vi "单板信息-new.vi"(8 "状态 2":string caption="系统连接状态", 11 "VIC_Receive":refnum<vi>) -> ()   [LabVIEW 2013]
panel:
  in  "偏差":dbl=10.0 format="%#.0f"
  in  "温度基准":dbl=25.0 caption="基准" format="%#.0f"
  in  "布尔 2":bool caption="判定"
  in  "偏差 2":dbl=0.05 caption="偏差" format="%.3f"
  in  "电压基准":dbl=3.7 format="%.3f"
  in  "布尔":bool caption="判定"
  out "电池充满标志位":string="是"
  out "电池运行状态":string="00"
  in  "从板板号 2":u8=1 caption="从板板号" min=1 max=30
  out "滑动杆":dbl(slide)=90.0 caption="SOC" scale=0.0..100.0 scale format="%#_6f"
  out "5":T1
  out "4":T2
  out "3":T3
  out "2":T4
  out "平均电流(A)":dbl
  out "外总压(V)":dbl
  out "总电流(A)":dbl
  out "协议是否公开":string="是"
  out "波特率":string="500Kbps"
  out "应用类型":string
  out "协议版本号":string
  out "SOH":dbl(slide)=30.0 scale=0.0..100.0 scale format="%#_6f"
  in  "刷新":bool
  in  "布尔 3":bool
  out "故障信息":string
  out "最小内阻位置":i32
  out "最大内阻位置":i32
  out "最小内阻":dbl
  out "最大内阻":dbl
  out "最低温度位置":i32
  out "最高温度位置":i32
  out "最低温度":dbl
  out "最高温度":dbl
  out "最低电压位置":i32
  out "最高电压位置":i32
  out "最低电压":dbl
  out "最高电压":dbl
  in  "主界面选项":enum32{"单选选项1", "单选选项2", "单选选项2 2"}(radio)
  in  "继电器状态 2":string[][](table)=[["RL1_ST", "", "RL5_ST"], ["RL2_ST", "", "RL6_ST"], ["RL3_ST", "", "RL7_ST"], ["RL4_ST", "", "RL8_ST"]]
  out "快换帧":T5
  out "从板参数":T6={"总电压"=0.0, "总电流"=0.0, "外总压"=0.0, "平均电流"=0.0, "SOC"=60.0, "SOH"=60.0, "最高电压"=0.0, "位置"=0.0, "最低电压"=0.0, "位置"=0.0, "压差"=0.0, "最高温度"=0.0, "位置"=0.0, "最低温度"=0.0, "位置"=0.0, "最大内阻"=0.0, "位置"=0.0, "最小内阻"=0.0, "位置"=0.0, "故障信息"="", "协议版本号"="", "应用类型"="", "波特率"="", "协议是否公开"="", "电池运行状态"="", "电池充满标志位"="", "Life:"=25.0} {"SOH" scale=0.0..100.0 scale format="%#.0f"; "SOC" scale=0.0..100.0 scale format="%#.0f"}
  out "Life:":dbl=25.0
  out "状态":bool
  out "高压板参数":T7={"总电压"=0.0, "总电流"=0.0, "外总压"=0.0, "平均电流"=0.0, "功率"=0.0, "总充电安时"=0.0, "总放电安时"=0.0, "故障信息"="", "协议版本号"="", "应用类型"="", "波特率"="", "协议是否公开"="", "电池运行状态"="", "Life:"=25.0, "正绝缘电阻"=0.0, "负绝缘电阻"=0.0} {"负绝缘电阻" format="%#.0f"; "正绝缘电阻" format="%#.0f"; "总放电安时" format="%#.0f"; "总充电安时" format="%#.0f"}
  out "继电器颜色":u32[](array[colorbox])
  out "继电器状态":string[](array[string])
  in  "选项卡控件":enum32{"从板监控", "从板信息2", "电压温度", "高压板监控"}(tab)=enum."从板信息2"
  out "从板参数":T8={"最高电压"=0.0, "位置1"=0.0, "最低电压"=0.0, "位置2"=0.0, "压差"=0.0, "最高温度"=0.0, "位置3"=0.0, "最低温度"=0.0, "位置4"=0.0, "温差"=0.0, "最高内阻"=0.0, "位置5"=0.0, "最低内阻"=0.0, "位置6"=0.0, "故障信息"="00", "最大充电总电压"=0.0, "最大充电电流"=0.0, "充电总安时"=0.0, "SOH 2"=0.0, "RL1_ST(fan)"="", "RL2_ST(heat)"="", "RL3_ST"="", "RL4_ST"="", "RL5_ST"="", "RL6_ST"="", "RL7_ST"="", "RL8_ST"=""}
  out "总电压(V)":dbl
  out "硬件故障":string[][](array[string])
  in  "欠压":u16(ring)
  in  "过压":u16(ring)
  in  "无效":u16(ring)
  in  "故障":u16(ring)
  in  "正常":u16(ring)
  out "供电电源电压(V)":string="0"
  out "内网总线负载率":string="0"
  out "供电电源状态":u16(ring)=1
  out "Flash存储器状态":u16(ring)
  out "外部EE存储器状态":u16(ring)=1
  out "内部EE存储器状态":u16(ring)=3
  out "系统时钟状态":u16(ring)
  out "内部总电压检测模块状态":u16(ring)
  out "外部总电压检测模块状态":u16(ring)
  out "绝缘检测模块状态":u16(ring)
  out "电流模块模块状态":u16(ring)=1 caption="电流检测模块状态"
  out "电池充电均衡模块状态":u16(ring)
  out "电池放电均衡模块状态":u16(ring)=1
  out "温度模块检测状态":u16(ring)=3 caption="温度检测模块状态"
  out "电压模块检测状态":u16(ring) caption="电压检测模块状态"
  out "1":T9 {"第12串" format="%#.2f"; "第11串" format="%#.2f"; "第10串" format="%#.2f"; "第9串" format="%#.2f"; "第8串" format="%#.2f"; "第7串" format="%#.2f"; "第6串" format="%#.2f"; "第5串" format="%#.2f"; "第4串" format="%#.2f"; "第3串" format="%#.2f"; "第2串" format="%#.2f"; "第1串" format="%#.2f"}
  out "1 7":T1 {"第60串" format="%.3f"; "第59串" format="%.3f"; "第58串" format="%.3f"; "第57串" format="%.3f"; "第56串" format="%.3f"; "第55串" format="%.3f"; "第54串" format="%.3f"; "第53串" format="%.3f"; "第52串" format="%.3f"; "第51串" format="%.3f"; "第50串" format="%.3f"; "第49串" format="%.3f"}
  out "1 6":T2 {"第48串" format="%.3f"; "第47串" format="%.3f"; "第46串" format="%.3f"; "第45串" format="%.3f"; "第44串" format="%.3f"; "第43串" format="%.3f"; "第42串" format="%.3f"; "第41串" format="%.3f"; "第40串" format="%.3f"; "第39串" format="%.3f"; "第38串" format="%.3f"; "第37串" format="%.3f"}
  out "1 4":T3 {"第36串" format="%.3f"; "第35串" format="%.3f"; "第34串" format="%.3f"; "第33串" format="%.3f"; "第32串" format="%.3f"; "第31串" format="%.3f"; "第30串" format="%.3f"; "第29串" format="%.3f"; "第28串" format="%.3f"; "第27串" format="%.3f"; "第26串" format="%.3f"; "第25串" format="%.3f"}
  out "1 3":T4 {"第24串" format="%.3f"; "第23串" format="%.3f"; "第22串" format="%.3f"; "第21串" format="%.3f"; "第20串" format="%.3f"; "第19串" format="%.3f"; "第18串" format="%.3f"; "第17串" format="%.3f"; "第16串" format="%.3f"; "第15串" format="%.3f"; "第14串" format="%.3f"; "第13串" format="%.3f"}
  out "1 102":T9 {"第12串" format="%.3f"; "第11串" format="%.3f"; "第10串" format="%.3f"; "第9串" format="%.3f"; "第8串" format="%.3f"; "第7串" format="%.3f"; "第6串" format="%.3f"; "第5串" format="%.3f"; "第4串" format="%.3f"; "第3串" format="%.3f"; "第2串" format="%.3f"; "第1串" format="%.3f"}
  out "高压板监控":T10={"总电压"=0.0, "总电流"=0.0, "外总压"=0.0, "平均电流"=0.0, "功率"=0.0, "总充电安时"=0.0, "总放电安时"=0.0, "正绝缘电阻"=0.0, "负绝缘电阻"=0.0, "版本协议号"="V1.2.34", "应用类型"="纯电动", "波特率"="500Kbps", "协议是否公开"="是", "故障信息"="00", "电池运行情况"="00"}
  in  "VCI_Receive":T11 {"Rsv3" max=0 format="%x"; "Rsv2" min=101 format="%x"; "Rsv1" format="%x"; "Data8" format="%x"; "Data7" format="%x"; "Data6" format="%x"; "Data5" format="%x"; "Data4" format="%x"; "Data3" format="%x"; "Data2" format="%x"; "Data1" format="%x"; "DataLen" format="%x"; "ExternFlag" format="%x"; "RemoteFlag" format="%x"; "SendType" format="%x"; "TimeFlag" format="%x"; "TimeStamp" format="%x"; "ID" format="%x"}
  in  "停止":bool
  out "单选选项2":bool
  # "Change frame"
  # "从板继电器"
  # "图例"
  # "单体电压(V)"
  # "温度(℃)"
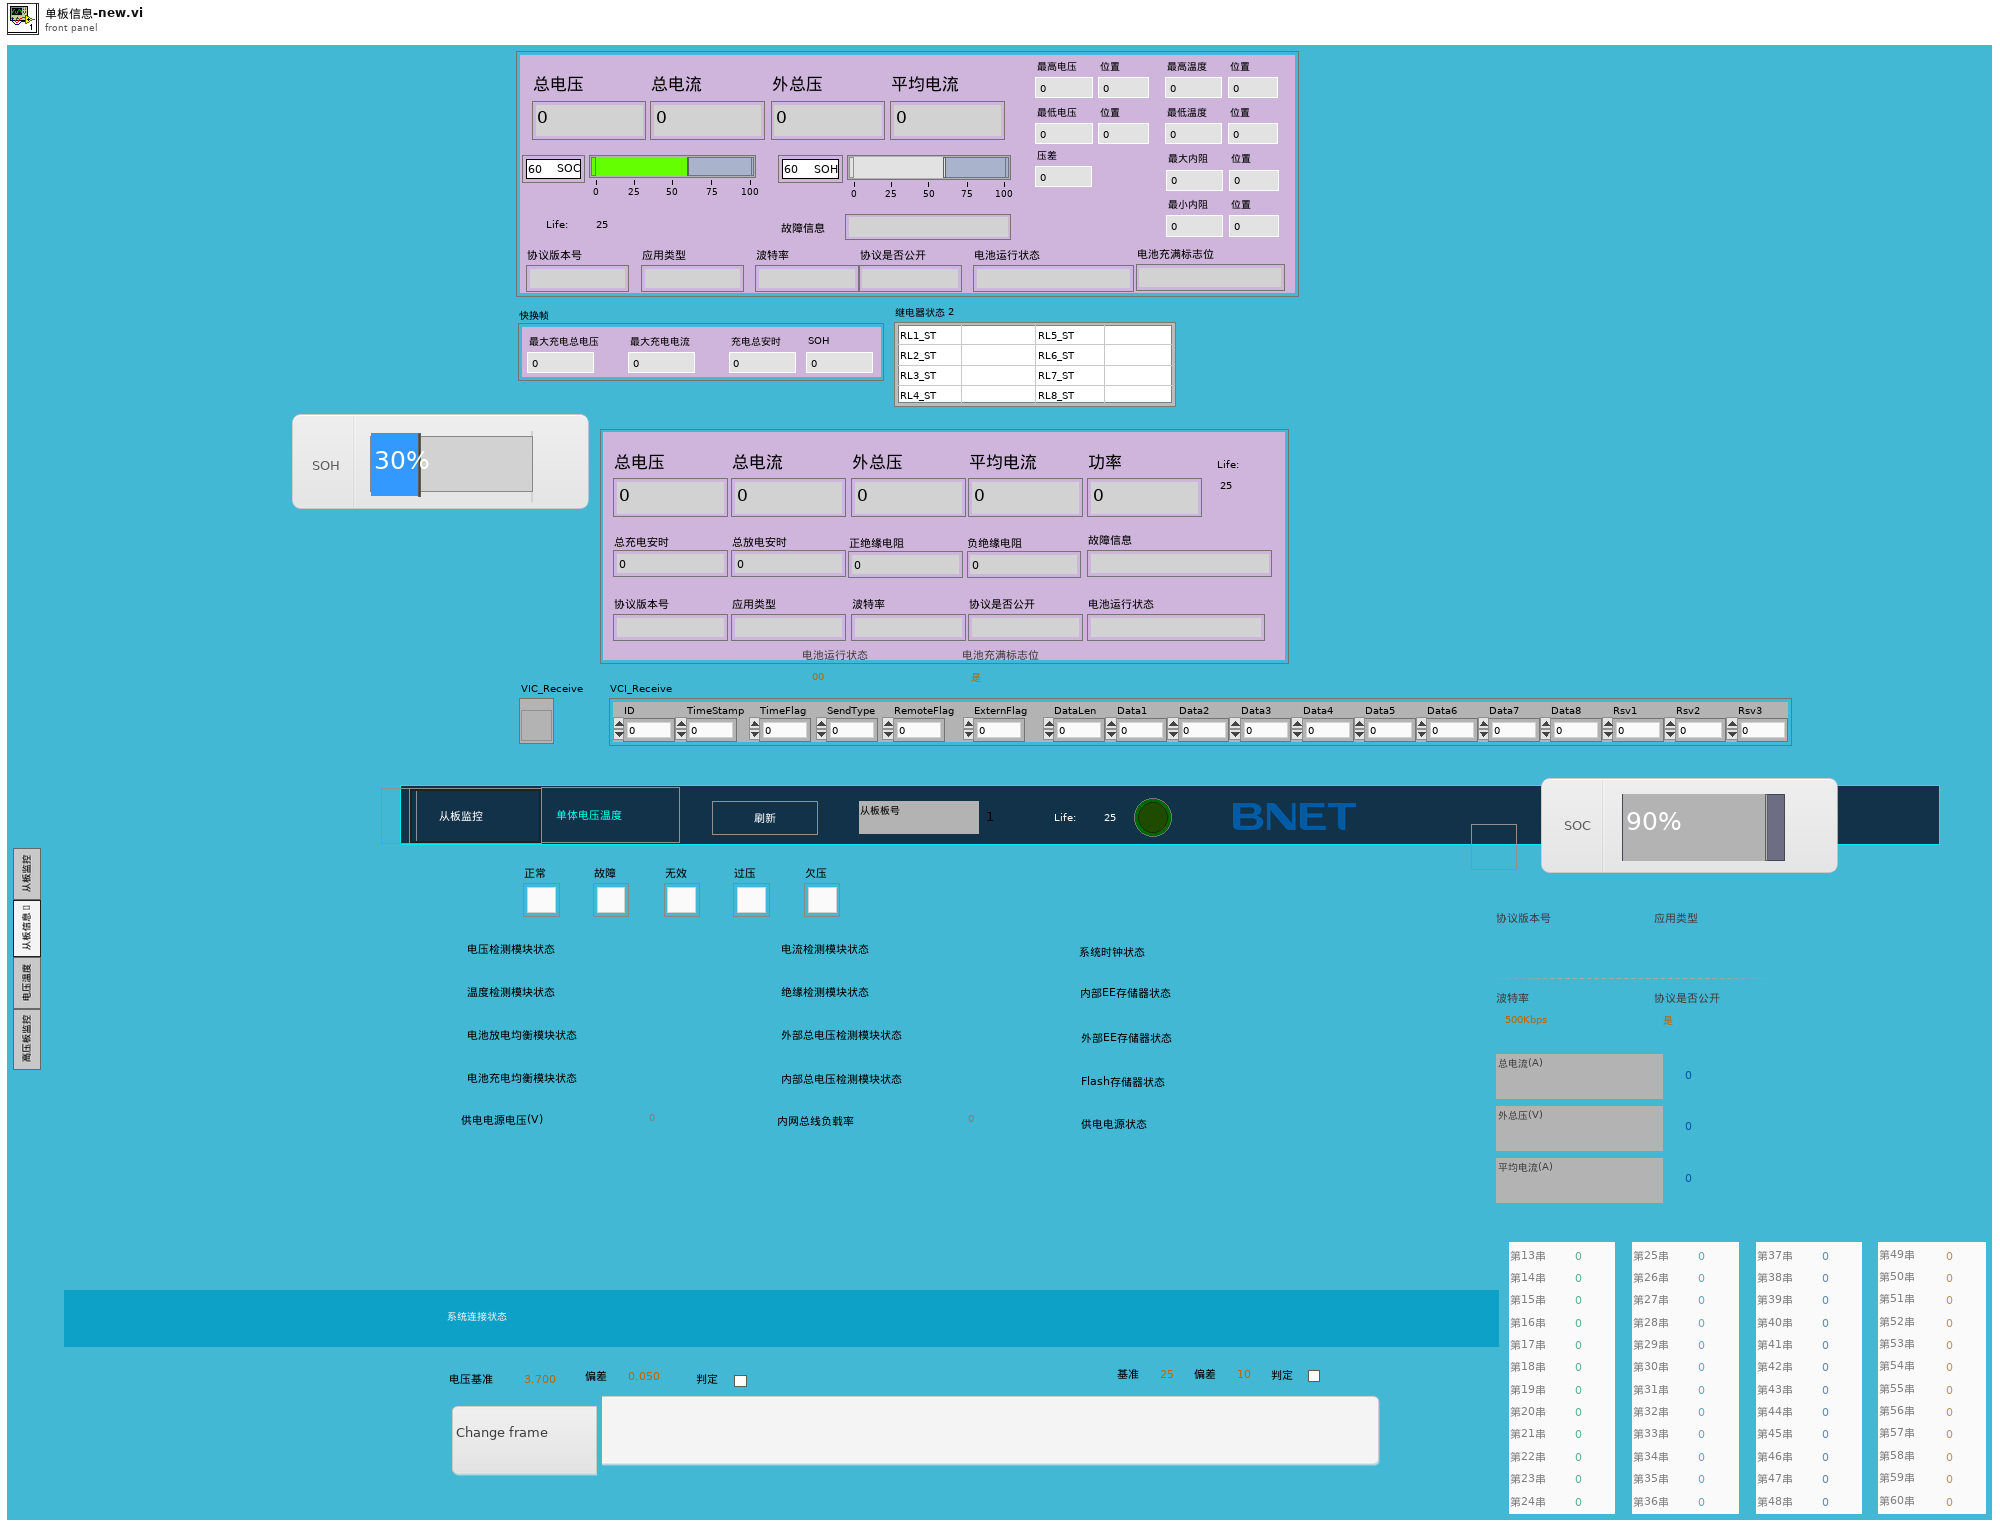
[diagram p1: front panel]
types:
  T1 = cluster{"第49串":dbl, "第50串":dbl, "第51串":dbl, "第52串":dbl, "第53串":dbl, "第54串":dbl, "第55串":dbl, "第56串":dbl, "第57串":dbl, "第58串":dbl, "第59串":dbl, "第60串":dbl}
  T2 = cluster{"第37串":dbl, "第38串":dbl, "第39串":dbl, "第40串":dbl, "第41串":dbl, "第42串":dbl, "第43串":dbl, "第44串":dbl, "第45串":dbl, "第46串":dbl, "第47串":dbl, "第48串":dbl}
  T3 = cluster{"第25串":dbl, "第26串":dbl, "第27串":dbl, "第28串":dbl, "第29串":dbl, "第30串":dbl, "第31串":dbl, "第32串":dbl, "第33串":dbl, "第34串":dbl, "第35串":dbl, "第36串":dbl}
  T4 = cluster{"第13串":dbl, "第14串":dbl, "第15串":dbl, "第16串":dbl, "第17串":dbl, "第18串":dbl, "第19串":dbl, "第20串":dbl, "第21串":dbl, "第22串":dbl, "第23串":dbl, "第24串":dbl}
  T5 = cluster{"SOH":dbl, "充电总安时":dbl, "最大充电电流":dbl, "最大充电总电压":dbl}
  T6 = cluster{"总电压":dbl, "总电流":dbl, "外总压":dbl, "平均电流":dbl, "SOC":dbl, "SOH":dbl, "最高电压":dbl, "位置":dbl, "最低电压":dbl, "位置":dbl, "压差":dbl, "最高温度":dbl, "位置":dbl, "最低温度":dbl, "位置":dbl, "最大内阻":dbl, "位置":dbl, "最小内阻":dbl, "位置":dbl, "故障信息":string, "协议版本号":string, "应用类型":string, "波特率":string, "协议是否公开":string, "电池运行状态":string, "电池充满标志位":string, "Life:":dbl}
  T7 = cluster{"总电压":dbl, "总电流":dbl, "外总压":dbl, "平均电流":dbl, "功率":dbl, "总充电安时":dbl, "总放电安时":dbl, "故障信息":string, "协议版本号":string, "应用类型":string, "波特率":string, "协议是否公开":string, "电池运行状态":string, "Life:":dbl, "正绝缘电阻":dbl, "负绝缘电阻":dbl}
  T8 = cluster{"最高电压":dbl, "位置1":dbl, "最低电压":dbl, "位置2":dbl, "压差":dbl, "最高温度":dbl, "位置3":dbl, "最低温度":dbl, "位置4":dbl, "温差":dbl, "最高内阻":dbl, "位置5":dbl, "最低内阻":dbl, "位置6":dbl, "故障信息":string, "最大充电总电压":dbl, "最大充电电流":dbl, "充电总安时":dbl, "SOH 2":dbl, "RL1_ST(fan)":string, "RL2_ST(heat)":string, "RL3_ST":string, "RL4_ST":string, "RL5_ST":string, "RL6_ST":string, "RL7_ST":string, "RL8_ST":string}
  T9 = cluster{"第1串":dbl, "第2串":dbl, "第3串":dbl, "第4串":dbl, "第5串":dbl, "第6串":dbl, "第7串":dbl, "第8串":dbl, "第9串":dbl, "第10串":dbl, "第11串":dbl, "第12串":dbl}
  T10 = cluster{"总电压":dbl, "总电流":dbl, "外总压":dbl, "平均电流":dbl, "功率":dbl, "总充电安时":dbl, "总放电安时":dbl, "正绝缘电阻":dbl, "负绝缘电阻":dbl, "版本协议号":string, "应用类型":string, "波特率":string, "协议是否公开":string, "故障信息":string, "电池运行情况":string}
  T11 = cluster{"ID":u32, "TimeStamp":u32, "TimeFlag":u8, "SendType":u8, "RemoteFlag":u8, "ExternFlag":u8, "DataLen":u8, "Data1":u8, "Data2":u8, "Data3":u8, "Data4":u8, "Data5":u8, "Data6":u8, "Data7":u8, "Data8":u8, "Rsv1":u8, "Rsv2":u8, "Rsv3":u8}
  T12 = cluster{dbl, dbl, dbl, dbl, dbl, dbl, dbl, dbl, dbl, dbl, dbl, dbl, dbl, dbl, "故障信息":string, dbl, dbl, dbl, dbl, "RL1_ST":string, "RL2_ST":string, "RL3_ST":string, "RL4_ST":string, "RL5_ST":string, "RL6_ST":string, "RL7_ST":string, "RL8_ST":string}
  T13 = enum32{"Invalid", "Standard", "Closed", "Hidden", "Minimized", "Maximized"}
  T14 = cluster{"[0]":u8, "[1]":u8, "[2]":u8, "[3]":u8, "[4]":u8, "[5]":u8, "[6]":u8, "[7]":u8, "[8]":u8, "[9]":u8, "[10]":u8, "[11]":u8}
  T15 = cluster{"[0]":dbl, "[1]":dbl, "[2]":dbl, "[3]":dbl, "[4]":dbl, "[5]":dbl, "[6]":dbl, "[7]":dbl, "[8]":dbl, "[9]":dbl, "[10]":dbl, "[11]":dbl}
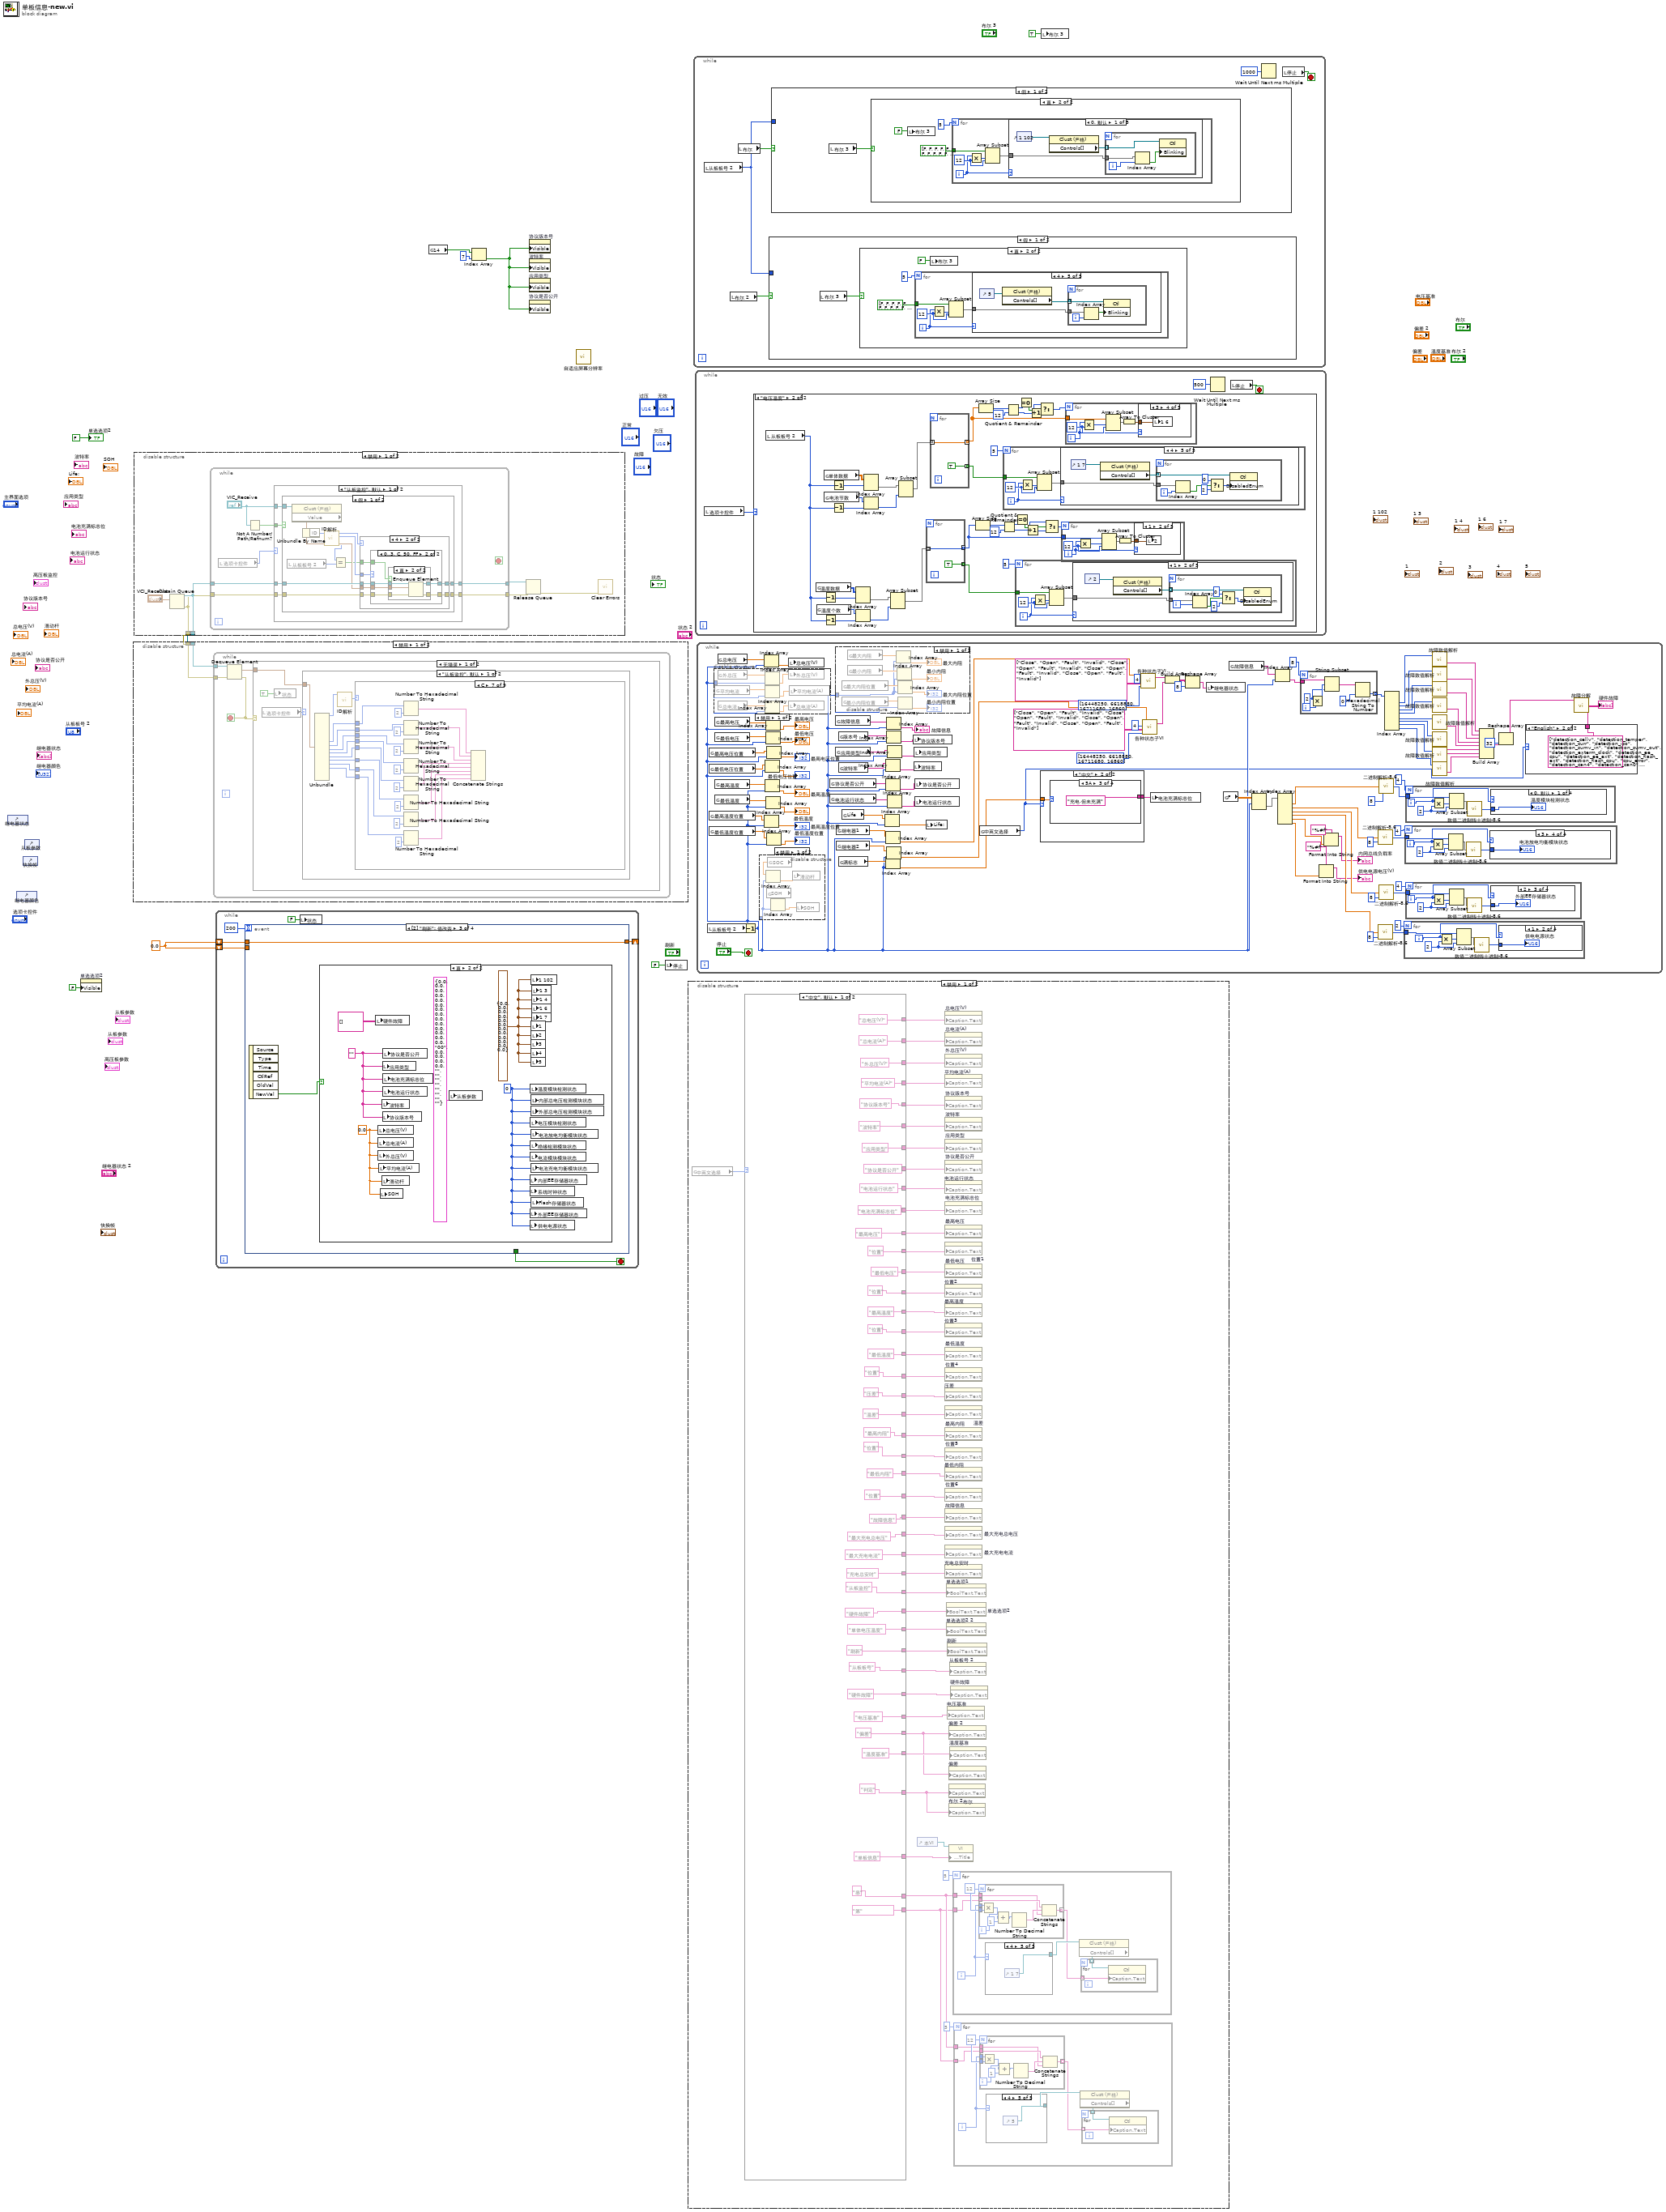
[diagram p0: block diagram]
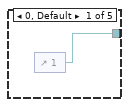
[diagram p2: hidden frame]
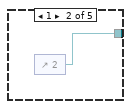
[diagram p3: hidden frame]
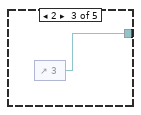
[diagram p4: hidden frame]
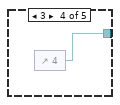
[diagram p5: hidden frame]
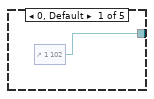
[diagram p6: hidden frame]
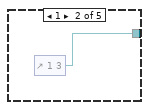
[diagram p7: hidden frame]
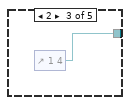
[diagram p8: hidden frame]
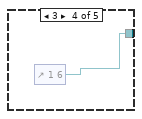
[diagram p9: hidden frame]
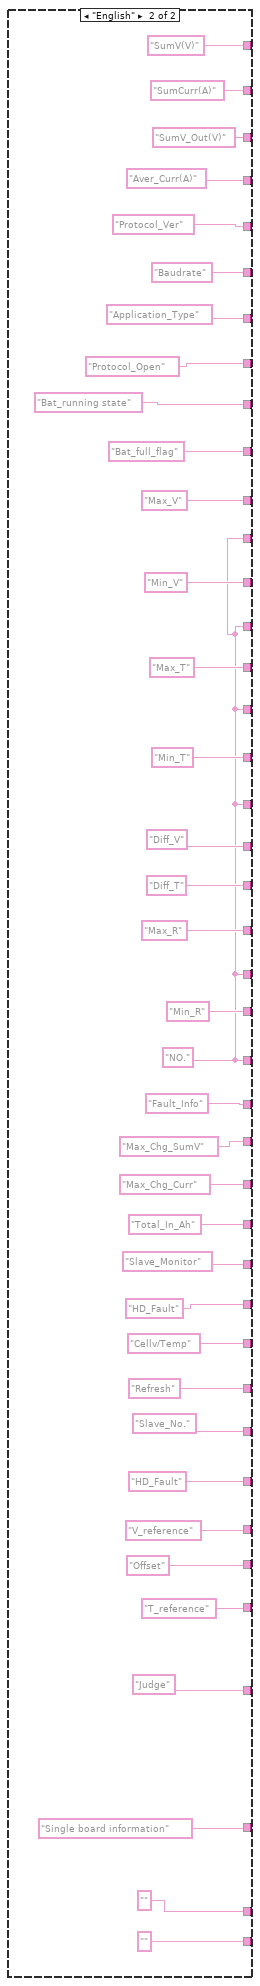
[diagram p10: hidden frame]
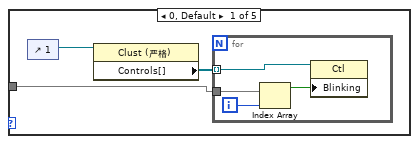
[diagram p13: hidden frame]
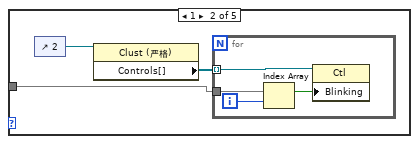
[diagram p14: hidden frame]
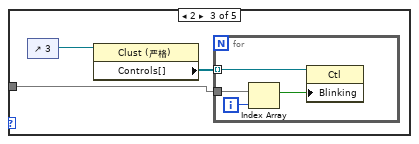
[diagram p15: hidden frame]
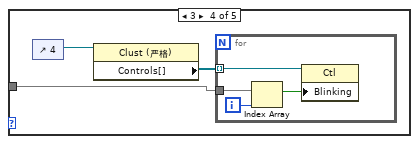
[diagram p16: hidden frame]
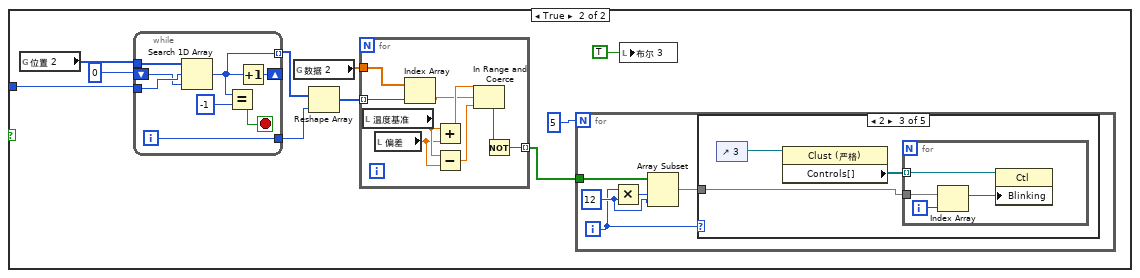
[diagram p17: hidden frame]
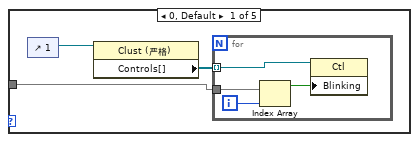
[diagram p18: hidden frame]
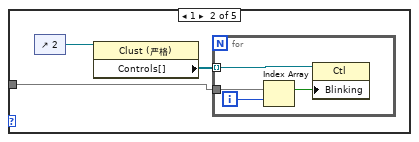
[diagram p19: hidden frame]
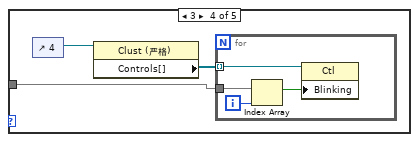
[diagram p20: hidden frame]
diagram:
  w5 = 0.0 ("Life:")
  n1 = control-ref of="继电器状态"() -> ()  [unwired: 1 out]
  n2 = control-ref of="继电器颜色"() -> ()  [unwired: 1 out]
  n3 = control-ref of="快换帧"() -> ()  [unwired: 1 out]
  n4 = control-ref of="从板参数"() -> ()  [unwired: 1 out]
  n5 = property on="单选选项2" class="Bool (严格)"("Visible"=FALSE ("可见")) -> ()  [unwired: 2 in, 2 out]
  n6 = disable-structure shown="禁用" {
    disable-tunnel: [w15 _] -> w10
    disable-tunnel: [w14 _] -> w9
    frame Disabled {
      n7 = Obtain Queue(element data type="VCI_Receive") -> (queue out=w15:refnum<queue>, error out=w14:errorcluster)  [unwired: 4 in, 1 out]
      n8 = while {
        tunnel: w15 -> [w22]
        tunnel: w14 -> [w21]
        tunnel: [w20] -> w13
        tunnel: [w19] -> w12
        stop <- w23 stop-if-true
        n9 = local read "选项卡控件"() -> (w17:enum32{"从板监控", "从板信息2", "电压温度", "高压板监控"})
        n10 = Not A Number/Path/Refnum?(number/path/refnum="VIC_Receive") -> (NaN/Path/Refnum?=w18:bool)
        n11 = case shown="\"从板监控\", 默认" w17 {
          tunnel: "VIC_Receive" -> [w30 w75]
          tunnel: w22 -> [w29 w74]
          tunnel: w21 -> [w28 w73]
          tunnel: [w27 w72] -> w20
          tunnel: [w26 w71] -> w19
          tunnel: w18 -> [w25 w70]
          frame "从板监控", Default {
            n12 = case shown="假" w25 {
              tunnel: w29 -> [w41 w69]
              tunnel: w28 -> [w40 w68]
              tunnel: [w38 w69] -> w27
              tunnel: [w37 w68] -> w26
              tunnel: w30 -> [w36 _]
              frame False {
                n13 = local read "从板板号 2"() -> (w31:u8)
                n14 = property class="Clust (严格)"(reference=w36) -> ("Value"=w39:T11)  [unwired: 1 in, 2 out]
                n15 = Unbundle By Name(w39) -> ("ID"=w42:u32)
                n16 = call "ID解析.vi"("ID"=w42) -> ("SA(4)"=w33:i32, "PF(2)"=w34:i32, "PDU(1)"=w35:i32)  [unwired: 8 out]
                n17 = Equal?(x=w33, y=w31) -> (x = y?=w32:bool)
                n18 = case shown="4" w35 {
                  tunnel: w41 -> [w44 w51]
                  tunnel: w40 -> [w43 w50]
                  tunnel: w39 -> [_ w49]
                  tunnel: [w44 w48] -> w38
                  tunnel: [w43 w47] -> w37
                  tunnel: w34 -> [_ w46]
                  tunnel: w32 -> [_ w45]
                  frame 0, Default {
                  }
                  frame 4 {
                    n19 = case shown="0..3, C, 50, FF" w46 {
                      tunnel: w51 -> [w53 w59]
                      tunnel: w50 -> [w52 w58]
                      tunnel: w49 -> [_ w57]
                      tunnel: [w53 w56] -> w48
                      tunnel: [w52 w55] -> w47
                      tunnel: w45 -> [_ w54]
                      frame 153, Default {
                      }
                      frame 0..3, 12, 80, 255 {
                        n20 = case shown="真" w54 {
                          tunnel: w59 -> [w61 w66]
                          tunnel: w58 -> [w60 w65]
                          tunnel: w57 -> [_ w64]
                          tunnel: [w61 w63] -> w56
                          tunnel: [w60 w62] -> w55
                          frame False {
                          }
                          frame True {
                            n21 = Enqueue Element(queue=w66, element=w64, error in (no error)=w65) -> (queue out=w63:refnum<queue>, error out=w62:errorcluster)  [unwired: 2 out]
                          }
                        }
                      }
                    }
                  }
                }
              }
              frame True {
                n22 = Wait Until Next ms Multiple(millisecond multiple=u32 100 ("毫秒倍数")) -> ()  [unwired: 1 out]
              }
            }
          }
          frame "高压板监控" {
            n23 = case shown="假" w70 {
              tunnel: w74 -> [w87 w115]
              tunnel: w73 -> [w86 w114]
              tunnel: [w84 w115] -> w72
              tunnel: [w83 w114] -> w71
              tunnel: w75 -> [w82 _]
              frame False {
                n24 = property class="Clust (严格)"(reference=w82) -> ("Value"=w85:T11)  [unwired: 1 in, 2 out]
                n25 = Unbundle By Name(w85) -> ("ID"=w88:u32)
                n26 = call "ID解析.vi"("ID"=w88) -> ("SA(4)"=w79:i32, "PF(2)"=w80:i32, "PDU(1)"=w81:i32)  [unwired: 8 out]
                n27 = Equal?(x=w79, y=62) -> (x = y?=w78:bool)
                n28 = case shown="4" w81 {
                  tunnel: w87 -> [w90 w97]
                  tunnel: w86 -> [w89 w96]
                  tunnel: w85 -> [_ w95]
                  tunnel: [w90 w94] -> w84
                  tunnel: [w89 w93] -> w83
                  tunnel: w80 -> [_ w92]
                  tunnel: w78 -> [_ w91]
                  frame 0, Default {
                  }
                  frame 4 {
                    n29 = case shown="0, 5, 8, C, FF" w92 {
                      tunnel: w97 -> [w99 w105]
                      tunnel: w96 -> [w98 w104]
                      tunnel: w95 -> [_ w103]
                      tunnel: [w99 w102] -> w94
                      tunnel: [w98 w101] -> w93
                      tunnel: w91 -> [_ w100]
                      frame 153, Default {
                      }
                      frame 0, 5, 8, 12, 255 {
                        n30 = case shown="真" w100 {
                          tunnel: w105 -> [w107 w112]
                          tunnel: w104 -> [w106 w111]
                          tunnel: w103 -> [_ w110]
                          tunnel: [w107 w109] -> w102
                          tunnel: [w106 w108] -> w101
                          frame False {
                          }
                          frame True {
                            n31 = Enqueue Element(queue=w112, element=w110, error in (no error)=w111) -> (queue out=w109:refnum<queue>, error out=w108:errorcluster)  [unwired: 2 out]
                          }
                        }
                      }
                    }
                  }
                }
                n32 = local write "状态"(FALSE ("接收")) -> ()
              }
              frame True {
                n33 = Wait Until Next ms Multiple(millisecond multiple=u32 100 ("毫秒倍数")) -> ()  [unwired: 1 out]
              }
            }
          }
        }
      }
      n34 = Release Queue(queue=w13, error in (no error)=w12) -> (error out=w11:errorcluster)  [unwired: 3 out]
      n35 = call <vilib>:"Clear Errors.vi"("error in (no error)"=w11) -> ()  [unwired: 7 out]
    }
    frame Enabled {
    }
  }
  n36 = disable-structure shown="禁用" {
    disable-tunnel: w10 -> [w117 _]
    disable-tunnel: w9 -> [w116 _]
    frame Disabled {
      n37 = while {
        tunnel: w117 -> [w120]
        tunnel: w116 -> [w119]
        stop <- w121 stop-if-true
        n38 = Dequeue Element(queue=w120, error in (no error)=w119) -> (element=w118:T11, error out=w121:errorcluster)  [unwired: 3 out]
        n39 = case shown="无错误" w121 {
          tunnel: w118 -> [w124 _]
          frame No Error {
            n40 = local read "选项卡控件"() -> (w123:enum32{"从板监控", "从板信息2", "电压温度", "高压板监控"})
            n41 = local write "状态"(TRUE ("接收")) -> ()
            n42 = case shown="\"从板监控\", 默认" w123 {
              tunnel: w124 -> [w135 w321]
              frame "从板监控", Default {
                n43 = Unbundle(w135) -> ("ID"=w134:u32, "Data1"=w132:u8, "Data2"=w131:u8, "Data3"=w130:u8, "Data4"=w129:u8, "Data5"=w128:u8, "Data6"=w127:u8, "Data7"=w126:u8, "Data8"=w125:u8)  [unwired: 9 out]
                n44 = call "ID解析.vi"("ID"=w134) -> ("PF(2)"=w133:i32)  [unwired: 10 out]
                n45 = case shown="C" w133 {
                  tunnel: w132 -> [_ w145 w174 w188 w210 w242 w262 w280 w285]
                  tunnel: w131 -> [_ w144 w173 w187 w209 w241 w261 _ w284]
                  tunnel: w130 -> [_ w143 w172 w186 w208 w240 w260 _ w283]
                  tunnel: w129 -> [_ w142 w171 w185 w207 w239 w259 _ _]
                  tunnel: w128 -> [_ w141 w170 w184 w206 w238 w258 _ w282]
                  tunnel: w127 -> [_ w140 w169 w183 w205 w237 w257 w279 _]
                  tunnel: w126 -> [_ w139 w156 w182 w204 w236 w256 _ _]
                  tunnel: w125 -> [_ w138 w155 _ w203 _ w255 _ w281]
                  frame 153, Default {
                    n46 = Wait Until Next ms Multiple(millisecond multiple=u32 2 ("毫秒倍数")) -> ()  [unwired: 1 out]
                  }
                  frame 0 {
                    n47 = Join Numbers(hi=w143, lo=w142) -> ((hi.lo)=w150:u16)
                    n48 = Join Numbers(hi=w141, lo=w140) -> ((hi.lo)=w152:u16)
                    n49 = Join Numbers(hi=w145, lo=w144) -> ((hi.lo)=w151:u16)
                    n50 = Join Numbers(hi=w139, lo=w138) -> ((hi.lo)=w146:u16)
                    n51 = call "输出分辨率计算.vi"("偏移量"=sgl -3000.0, "分辨率"=0.1, "数值 3"=w150, "数值 2"=w146) -> ()  [unwired: 2 in, 6 out]
                    n52 = call "输出分辨率计算.vi"("分辨率"=0.1, "数值 3"=w152, "数值 2"=w151) -> ("输出2"=w137:dbl)  [unwired: 3 in, 5 out]
                  }
                  frame 144 {
                    n53 = Join Numbers(hi=w172, lo=w171) -> ((hi.lo)=w178:u16)
                    n54 = Join Numbers(hi=w170, lo=w169) -> ((hi.lo)=w168:u16)
                    n55 = Join Numbers(hi=w174, lo=w173) -> ((hi.lo)=w179:u16)
                    n56 = call "二进制解析-8.6.vi"("索引"=8, "数值"=w156) -> ("低位子数组"=w159:i32[])  [unwired: 3 out]
                    n57 = call "二进制解析-8.6.vi"("索引"=4, "数值"=w155) -> ("高位子数组"=w158:i32[])  [unwired: 3 out]
                    n58 = Insert Into Array(array=w159, new element=w158) -> (w157:i32[])  [unwired: 1 in]
                    n59 = call "输出分辨率计算.vi"("分辨率"=0.001, "数值 2"=w168) -> ("输出2"=w162:dbl)  [unwired: 4 in, 5 out]
                    n60 = local read "快换帧"() -> (w166:T5)
                    n61 = call "数值二进制转十进制-8.6.vi"("子数组"=w157) -> ("十进制数值"=w154:i32)  [unwired: 4 out]
                    n62 = call "输出分辨率计算.vi"("分辨率"=0.1, "数值 3"=w154, "数值 2"=w179) -> ("输出3"=w153:dbl, "输出2"=w163:dbl)  [unwired: 3 in, 4 out]
                    n63 = call "输出分辨率计算.vi"("偏移量"=sgl -3000.0, "分辨率"=0.1, "数值 3"=w178) -> ("输出3"=w164:dbl)  [unwired: 3 in, 5 out]
                    n64 = Bundle(cluster=w166, "SOH"=w153, "充电总安时"=w162, "最大充电电流"=w164, "最大充电总电压"=w163) -> (w165:T5)
                    n65 = local write "快换帧"(w165) -> ()
                  }
                  frame 1 {
                    n66 = Join Numbers(hi=w188, lo=w187) -> ((hi.lo)=w189:u16)
                    n67 = Join Numbers(hi=w186, lo=w185) -> ((hi.lo)=w190:u16)
                    n68 = call "二进制解析-8.6.vi"("索引"=8, "数值"=w182) -> ("低位子数组"=w198:i32[])  [unwired: 3 out]
                    n69 = call "二进制解析-8.6.vi"("索引"=8, "数值"=w184) -> ("低位子数组"=w195:i32[])  [unwired: 3 out]
                    n70 = call "二进制解析-8.6.vi"("索引"=4, "数值"=w183) -> ("低位子数组"=w197:i32[], "高位子数组"=w196:i32[])  [unwired: 2 out]
                    n71 = Insert Into Array(array=w195, new element=w196) -> (w200:i32[])  [unwired: 1 in]
                    n72 = Insert Into Array(array=w197, new element=w198) -> (w199:i32[])  [unwired: 1 in]
                    n73 = call "输出分辨率计算.vi"("分辨率"=0.001, "数值 3"=w190, "数值 2"=w189) -> ("输出3"=w181:dbl, "输出2"=w180:dbl)  [unwired: 3 in, 4 out]
                    n74 = call "数值二进制转十进制-8.6.vi"("子数组"=w200) -> ()  [unwired: 5 out]
                    n75 = call "数值二进制转十进制-8.6.vi"("子数组"=w199) -> ()  [unwired: 5 out]
                  }
                  frame 2 {
                    n76 = call "二进制解析-8.6.vi"("索引"=8, "数值"=w203) -> ("低位子数组"=w224:i32[])  [unwired: 3 out]
                    n77 = call "二进制解析-8.6.vi"("索引"=8, "数值"=w205) -> ("低位子数组"=w227:i32[])  [unwired: 3 out]
                    n78 = call "二进制解析-8.6.vi"("索引"=4, "数值"=w204) -> ("低位子数组"=w225:i32[], "高位子数组"=w226:i32[])  [unwired: 2 out]
                    n79 = call "二进制解析-8.6.vi"("索引"=8, "数值"=w206) -> ("低位子数组"=w218:i32[])  [unwired: 3 out]
                    n80 = call "二进制解析-8.6.vi"("索引"=8, "数值"=w208) -> ("低位子数组"=w215:i32[])  [unwired: 3 out]
                    n81 = call "二进制解析-8.6.vi"("索引"=4, "数值"=w207) -> ("低位子数组"=w217:i32[], "高位子数组"=w216:i32[])  [unwired: 2 out]
                    n82 = call "输出分辨率计算.vi"("偏移量"=sgl -40.0, "分辨率"=1.0, "数值 3"=w209, "数值 2"=w210) -> ()  [unwired: 2 in, 6 out]
                    n83 = Insert Into Array(array=w227, new element=w226) -> (w222:i32[])  [unwired: 1 in]
                    n84 = Insert Into Array(array=w225, new element=w224) -> (w223:i32[])  [unwired: 1 in]
                    n85 = Insert Into Array(array=w215, new element=w216) -> (w220:i32[])  [unwired: 1 in]
                    n86 = Insert Into Array(array=w217, new element=w218) -> (w219:i32[])  [unwired: 1 in]
                    n87 = call "数值二进制转十进制-8.6.vi"("子数组"=w222) -> ("十进制数值"=w231:i32)  [unwired: 4 out]
                    n88 = call "数值二进制转十进制-8.6.vi"("子数组"=w220) -> ()  [unwired: 5 out]
                    n89 = call "数值二进制转十进制-8.6.vi"("子数组"=w223) -> ("十进制数值"=w232:i32)  [unwired: 4 out]
                    n90 = call "数值二进制转十进制-8.6.vi"("子数组"=w219) -> ()  [unwired: 5 out]
                    n91 = call "输出分辨率计算.vi"("分辨率"=0.1, "数值 3"=w232, "数值 2"=w231) -> ("输出3"=w201:dbl, "输出2"=w202:dbl)  [unwired: 3 in, 4 out]
                  }
                  frame 3 {
                    n92 = Join Numbers(hi=w242, lo=w241) -> ((hi.lo)=w243:u16)
                    n93 = Join Numbers(hi=w240, lo=w239) -> ((hi.lo)=w244:u16)
                    n94 = call "二进制解析-8.6.vi"("索引"=8, "数值"=w236) -> ("低位子数组"=w252:i32[])  [unwired: 3 out]
                    n95 = call "二进制解析-8.6.vi"("索引"=8, "数值"=w238) -> ("低位子数组"=w249:i32[])  [unwired: 3 out]
                    n96 = call "二进制解析-8.6.vi"("索引"=4, "数值"=w237) -> ("低位子数组"=w251:i32[], "高位子数组"=w250:i32[])  [unwired: 2 out]
                    n97 = Insert Into Array(array=w249, new element=w250) -> (w254:i32[])  [unwired: 1 in]
                    n98 = Insert Into Array(array=w251, new element=w252) -> (w253:i32[])  [unwired: 1 in]
                    n99 = call "输出分辨率计算.vi"("分辨率"=0.001, "数值 3"=w244, "数值 2"=w243) -> ("输出3"=w234:dbl, "输出2"=w235:dbl)  [unwired: 3 in, 4 out]
                    n100 = call "数值二进制转十进制-8.6.vi"("子数组"=w254) -> ()  [unwired: 5 out]
                    n101 = call "数值二进制转十进制-8.6.vi"("子数组"=w253) -> ()  [unwired: 5 out]
                  }
                  frame 12 {
                    n102 = Number To Hexadecimal String(1:i16 2 ("宽度(-)"), 2:w262) -> (0:w271:string)
                    n103 = Number To Hexadecimal String(1:i16 2 ("宽度(-)"), 2:w261) -> (0:w272:string)
                    n104 = Number To Hexadecimal String(1:i16 2 ("宽度(-)"), 2:w260) -> (0:w273:string)
                    n105 = Number To Hexadecimal String(1:i16 2 ("宽度(-)"), 2:w259) -> (0:w274:string)
                    n106 = Number To Hexadecimal String(1:i16 2 ("宽度(-)"), 2:w258) -> (0:w275:string)
                    n107 = Number To Hexadecimal String(1:i16 2 ("宽度(-)"), 2:w257) -> (0:w276:string)
                    n108 = Number To Hexadecimal String(1:i16 2 ("宽度(-)"), 2:w256) -> (0:w277:string)
                    n109 = Number To Hexadecimal String(1:i16 2 ("宽度(-)"), 2:w255) -> (0:w278:string)
                    n110 = Concatenate Strings(w271, w272, w273, w274, w275, w276, w277, w278) -> ()  [unwired: 1 out]
                  }
                  frame 80 {
                  }
                  frame 255 {
                    n111 = call "二进制解析-8.6.vi"("索引"=4, "数值"=w285) -> ("低位子数组"=w286:i32[], "高位子数组"=w287:i32[])  [unwired: 2 out]
                    n112 = call "二进制解析-8.6.vi"("索引"=6, "数值"=w284) -> ("低位子数组"=w297:i32[], "高位子数组"=w296:i32[])  [unwired: 2 out]
                    n113 = call "二进制解析-8.6.vi"("索引"=7, "数值"=w283) -> ("高位子数组"=w301:i32[])  [unwired: 3 out]
                    n114 = call "数值二进制转十进制-8.6.vi"("子数组"=w297) -> ("十进制数值"=w298:i32)  [unwired: 4 out]
                    n115 = call "数值二进制转十进制-8.6.vi"("子数组"=w286) -> ("十进制数值"=w289:i32)  [unwired: 4 out]
                    n116 = call "数值二进制转十进制-8.6.vi"("子数组"=w296) -> ("十进制数值"=w299:i32)  [unwired: 4 out]
                    n117 = call "数值二进制转十进制-8.6.vi"("子数组"=w301) -> ("十进制数值"=w302:i32)  [unwired: 4 out]
                    n118 = call "数值二进制转十进制-8.6.vi"("子数组"=w287) -> ("十进制数值"=w288:i32)  [unwired: 4 out]
                    n119 = case shown="1" w302 {
                      tunnel: ["不公开" "公开"] -> _
                      frame 0, Default {
                      }
                      frame 1 {
                      }
                    }
                    n120 = case shown="0, 默认" w298 {
                      tunnel: ["500Kps" "250Kps"] -> _
                      frame 0, Default {
                      }
                      frame 1 {
                      }
                    }
                    n121 = Number To Decimal String(number=w288) -> (decimal integer string=w290:string)  [unwired: 1 out]
                    n122 = case shown="4" w299 {
                      tunnel: [_ "纯电动BMS" "混合动力BMS" "储能" "快换"] -> _
                      frame 0, Default {
                      }
                      frame 1 {
                      }
                      frame 2 {
                      }
                      frame 3 {
                      }
                      frame 4 {
                      }
                    }
                    n123 = Number To Decimal String(number=w289) -> (decimal integer string=w292:string)  [unwired: 1 out]
                    n124 = call "运行模式解析.vi"("输入值"=w282) -> ()  [unwired: 1 in, 1 out]
                    n125 = Concatenate Strings("V" ("字符串"), w290, "." ("字符串"), w292) -> ()  [unwired: 1 out]
                  }
                }
              }
              frame "高压板监控" {
                n126 = Unbundle(w321) -> ("ID"=w320:u32, "Data1"=w318:u8, "Data2"=w317:u8, "Data3"=w316:u8, "Data4"=w315:u8, "Data5"=w314:u8, "Data6"=w313:u8, "Data7"=w312:u8, "Data8"=w311:u8)  [unwired: 9 out]
                n127 = call "ID解析.vi"("ID"=w320) -> ("PF(2)"=w319:i32)  [unwired: 10 out]
                n128 = case shown="99, 默认" w319 {
                  tunnel: w318 -> [_ w336 w355 w373 w401]
                  tunnel: w317 -> [_ w335 w354 w372 w400]
                  tunnel: w316 -> [_ w334 w353 w371 w399]
                  tunnel: w315 -> [_ w333 w352 w370 _]
                  tunnel: w314 -> [_ w332 w351 w369 w398]
                  tunnel: w313 -> [_ w331 w350 w368 _]
                  tunnel: w312 -> [_ w330 w349 w367 _]
                  tunnel: w311 -> [_ w329 w348 w366 w397]
                  frame 153, Default {
                    n129 = Wait Until Next ms Multiple(millisecond multiple=u32 2 ("毫秒倍数")) -> ()  [unwired: 1 out]
                  }
                  frame 0 {
                    n130 = Join Numbers(hi=w334, lo=w333) -> ((hi.lo)=w341:u16)
                    n131 = Join Numbers(hi=w332, lo=w331) -> ((hi.lo)=w343:u16)
                    n132 = Join Numbers(hi=w336, lo=w335) -> ((hi.lo)=w342:u16)
                    n133 = Join Numbers(hi=w330, lo=w329) -> ((hi.lo)=w337:u16)
                    n134 = call "输出分辨率计算.vi"("偏移量"=sgl -3000.0, "分辨率"=0.1, "数值 3"=w341, "数值 2"=w337) -> ("输出3"=w323:dbl, "输出2"=w324:dbl)  [unwired: 2 in, 4 out]
                    n135 = call "输出分辨率计算.vi"("分辨率"=0.1, "数值 3"=w343, "数值 2"=w342) -> ("输出3"=w325:dbl, "输出2"=w326:dbl)  [unwired: 3 in, 4 out]
                    n136 = local read "高压板监控"() -> (w328:T10)
                    n137 = Bundle By Name(cluster=w328, "总电压"=w326, "外总压"=w325, "平均电流"=w324, "总电流"=w323) -> (w327:T10)
                    n138 = local write "高压板监控"(w327) -> ()
                  }
                  frame 5 {
                    n139 = Join Numbers(hi=w355, lo=w354) -> ((hi.lo)=w358:u16)
                    n140 = Join Numbers(hi=w353, lo=w352) -> ((hi.lo)=w357:u16)
                    n141 = Join Numbers(hi=w351, lo=w350) -> ((hi.lo)=w359:u16)
                    n142 = Join Numbers(hi=w349, lo=w348) -> ((hi.lo)=w360:u16)
                    n143 = Join Numbers(hi=w358, lo=w357) -> ((hi.lo)=w362:u32)
                    n144 = Join Numbers(hi=w359, lo=w360) -> ((hi.lo)=w361:u32)
                    n145 = call "输出分辨率计算.vi"("分辨率"=0.001, "数值 3"=w361, "数值 2"=w362) -> ("输出3"=w345:dbl, "输出2"=w346:dbl)  [unwired: 3 in, 4 out]
                    n146 = local read "高压板监控"() -> (w347:T10)
                    n147 = Bundle By Name(cluster=w347, "总充电安时"=w346, "总放电安时"=w345) -> (w344:T10)
                    n148 = local write "高压板监控"(w344) -> ()
                  }
                  frame 12 {
                    n149 = Number To Hexadecimal String(1:i16 2 ("宽度(-)"), 2:w373) -> (0:w382:string)
                    n150 = Number To Hexadecimal String(1:i16 2 ("宽度(-)"), 2:w372) -> (0:w383:string)
                    n151 = Number To Hexadecimal String(1:i16 2 ("宽度(-)"), 2:w371) -> (0:w384:string)
                    n152 = Number To Hexadecimal String(1:i16 2 ("宽度(-)"), 2:w370) -> (0:w385:string)
                    n153 = Number To Hexadecimal String(1:i16 2 ("宽度(-)"), 2:w369) -> (0:w386:string)
                    n154 = Number To Hexadecimal String(1:i16 2 ("宽度(-)"), 2:w368) -> (0:w387:string)
                    n155 = Number To Hexadecimal String(1:i16 2 ("宽度(-)"), 2:w367) -> (0:w388:string)
                    n156 = Number To Hexadecimal String(1:i16 2 ("宽度(-)"), 2:w366) -> (0:w389:string)
                    n157 = Concatenate Strings(w382, w383, w384, w385, w386, w387, w388, w389) -> (w364:string)
                    n158 = local read "高压板监控"() -> (w365:T10)
                    n159 = Bundle By Name(cluster=w365, "故障信息"=w364) -> (w363:T10)
                    n160 = local write "高压板监控"(w363) -> ()
                  }
                  frame 255 {
                    n161 = local write "Life:"(w397) -> ()
                    n162 = call "二进制解析-8.6.vi"("索引"=4, "数值"=w401) -> ("低位子数组"=w402:i32[], "高位子数组"=w403:i32[])  [unwired: 2 out]
                    n163 = call "二进制解析-8.6.vi"("索引"=6, "数值"=w400) -> ("低位子数组"=w413:i32[], "高位子数组"=w412:i32[])  [unwired: 2 out]
                    n164 = call "二进制解析-8.6.vi"("索引"=7, "数值"=w399) -> ("高位子数组"=w417:i32[])  [unwired: 3 out]
                    n165 = call "数值二进制转十进制-8.6.vi"("子数组"=w413) -> ("十进制数值"=w414:i32)  [unwired: 4 out]
                    n166 = call "数值二进制转十进制-8.6.vi"("子数组"=w402) -> ("十进制数值"=w405:i32)  [unwired: 4 out]
                    n167 = call "数值二进制转十进制-8.6.vi"("子数组"=w412) -> ("十进制数值"=w415:i32)  [unwired: 4 out]
                    n168 = call "数值二进制转十进制-8.6.vi"("子数组"=w417) -> ("十进制数值"=w418:i32)  [unwired: 4 out]
                    n169 = call "数值二进制转十进制-8.6.vi"("子数组"=w403) -> ("十进制数值"=w404:i32)  [unwired: 4 out]
                    n170 = case shown="1" w418 {
                      tunnel: ["不公开" "公开"] -> w392
                      frame 0, Default {
                      }
                      frame 1 {
                      }
                    }
                    n171 = case shown="0, 默认" w414 {
                      tunnel: ["500Kps" "250Kps"] -> w393
                      frame 0, Default {
                      }
                      frame 1 {
                      }
                    }
                    n172 = Number To Decimal String(number=w404) -> (decimal integer string=w406:string)  [unwired: 1 out]
                    n173 = case shown="4" w415 {
                      tunnel: [_ "纯电动BMS" "混合动力BMS" "储能" "快换"] -> w394
                      frame 0, Default {
                      }
                      frame 1 {
                      }
                      frame 2 {
                      }
                      frame 3 {
                      }
                      frame 4 {
                      }
                    }
                    n174 = Number To Decimal String(number=w405) -> (decimal integer string=w408:string)  [unwired: 1 out]
                    n175 = call "运行模式解析.vi"("输入值"=w398) -> ("输出值"=w391:string)  [unwired: 1 in]
                    n176 = Concatenate Strings("V" ("字符串"), w406, "." ("字符串"), w408) -> (w395:string)
                    n177 = local read "高压板监控"() -> (w396:T10)
                    n178 = Bundle By Name(cluster=w396, "版本协议号"=w395, "应用类型"=w394, "波特率"=w393, "协议是否公开"=w392, "电池运行情况"=w391) -> (w390:T10)
                    n179 = local write "高压板监控"(w390) -> ()
                  }
                }
              }
            }
          }
          frame Error {
            n180 = Wait Until Next ms Multiple(millisecond multiple=u32 100 ("毫秒倍数")) -> ()  [unwired: 1 out]
          }
        }
      }
    }
    frame Enabled {
    }
  }
  n181 = while {
    shift-right: [w431] -> _
    shift-left: w5 -> [w430]
    shift-left: w5 -> [w429]
    stop <- w432 stop-if-true
    n182 = event shown="[2] \"刷新\": 值改变" {
      selector: _ -> [_ _ _ _]
      dyn-events: _ -> [_ _ _ _]
      timeout: 200 -> [_ _ _ _]
      tunnel: [_ _ _ w519] -> w432
      tunnel: [w437 w500 w511 w518] -> w431
      tunnel: w430 -> [w436 w500 w511 w518]
      tunnel: w429 -> [w435 _ _ _]
      event Timeout {
        n183 = event-data() -> ()  [unwired: 3 out]
        n184 = control-ref of="单选选项2 2"() -> (w439:refnum<vi>)
        n185 = control-ref of="单选选项2"() -> (w446:refnum<vi>)
        n186 = control-ref of="单选选项1"() -> (w447:refnum<vi>)
        n187 = local read "主界面选项"() -> (w448:enum32{"单选选项1", "单选选项2", "单选选项2 2"})
        n188 = Not Equal?(x=w436, y=w435) -> (x != y?=w434:bool)
        n189 = Build Array(w447, w446, w439) -> (w445:refnum<vi>[])
        n190 = local write "状态"(w434) -> ()
        n191 = case shown="\"单选选项2\"" w448 {
          selector: w448 -> [w483 w490 w496]
          tunnel: w445 -> [w484 w493 w499]
          tunnel: [w482 w492 w498] -> w442
          tunnel: [w481 w491 w497] -> w441
          tunnel: [TRUE TRUE TRUE] -> w440
          tunnel: [enum32{"从板监控", "从板信息2", "电压温度", "高压板监控"}."从板监控" ("选项卡控件") enum32{"从板监控", "从板信息2", "电压温度", "高压板监控"}."从板信息2" ("选项卡控件") enum32{"从板监控", "从板信息2", "电压温度", "高压板监控"}."电压温度" ("选项卡控件")] -> w438
          frame "单选选项1", Default {
            n192 = local read "继电器状态"() -> (w487:string[])
            n193 = local read "快换帧"() -> (w486:T5)
            n194 = local read "最高电压位置"() -> (w462:i32)
            n195 = local read "最低电压位置"() -> (w461:i32)
            n196 = local read "最高温度位置"() -> (w458:i32)
            n197 = local read "最低温度位置"() -> (w457:i32)
            n198 = local read "最大内阻位置"() -> (w455:i32)
            n199 = local read "最小内阻位置"() -> (w453:i32)
            n200 = local read "最高电压"() -> (w464:dbl)
            n201 = local read "最低电压"() -> (w463:dbl)
            n202 = local read "最高温度"() -> (w460:dbl)
            n203 = local read "最低温度"() -> (w459:dbl)
            n204 = local read "最大内阻"() -> (w456:dbl)
            n205 = local read "最小内阻"() -> (w454:dbl)
            n206 = local read "故障信息"() -> (w466:string)
            n207 = Index Array(array=w487) -> (element #1=w475:string, element #2=w474:string, element #3=w473:string, element #4=w472:string, element #5=w471:string, element #6=w470:string, element #7=w469:string, element #8=w468:string)  [unwired: 8 in]
            n208 = Unbundle(w486) -> ("SOH"=w451:dbl, "充电总安时"=w479:dbl, "最大充电电流"=w478:dbl, "最大充电总电压"=w477:dbl)
            n209 = Delete From Array(array=w484, index=w483) -> (deleted portion=w481:refnum<vi>, array with subset deleted=w482:refnum<vi>[])  [unwired: 1 in]
            n210 = local read "从板参数"() -> (w476:T8)
            n211 = Subtract(x=w464, y=w463) -> (x-y=w465:dbl)
            n212 = Subtract(x=w460, y=w459) -> (x-y=w480:dbl)
            n213 = Bundle(cluster=w476, "最高电压"=w464, "位置1"=w462, "最低电压"=w463, "位置2"=w461, "压差"=w465, "最高温度"=w460, "位置3"=w458, "最低温度"=w459, "位置4"=w457, "温差"=w480, "最高内阻"=w456, "位置5"=w455, "最低内阻"=w454, "位置6"=w453, "故障信息"=w466, "最大充电总电压"=w477, "最大充电电流"=w478, "充电总安时"=w479, "SOH 2"=w451, "RL1_ST(fan)"=w475, "RL2_ST(heat)"=w474, "RL3_ST"=w473, "RL4_ST"=w472, "RL5_ST"=w471, "RL6_ST"=w470, "RL7_ST"=w469, "RL8_ST"=w468) -> (w485:T8)
            n214 = local write "从板参数"(w485) -> ()
          }
          frame "单选选项2" {
            n215 = Delete From Array(array=w493, index=w490) -> (deleted portion=w491:refnum<vi>, array with subset deleted=w492:refnum<vi>[])  [unwired: 1 in]
          }
          frame "单选选项2 2" {
            n216 = Delete From Array(array=w499, index=w496) -> (deleted portion=w497:refnum<vi>, array with subset deleted=w498:refnum<vi>[])  [unwired: 1 in]
          }
        }
        n217 = for {
          tunnel: w442 -> [w450] mode=indexing
          tunnel: u32 16777215 -> [w449]
          n218 = property class="Bool (严格)"(reference=w450, "BoolText.TextColor"=w449) -> ()  [unwired: 1 in, 2 out]
        }
        n219 = property class="Bool (严格)"(reference=w441, "BoolText.TextColor"=u32 65511) -> ()  [unwired: 1 in, 2 out]
        n220 = local write "选项卡控件"(w438) -> ()
        n221 = property on="从板板号 2" class="DigNum (严格)"("Visible"=w440) -> ()  [unwired: 2 in, 2 out]
        n222 = local read "Life:"() -> (w437:dbl)
      }
      event "从板板号 2": Value Change {
        n223 = event-data() -> ("OldVal"=w503:u8, "NewVal"=w502:u8)  [unwired: 5 out]
        n224 = Not Equal?(x=w503, y=w502) -> (x != y?=w501:bool)
        n225 = case shown="真" w501 {
          frame False {
          }
          frame True {
            w504 = 0
            w506 = T9 {"第1串"=0.0, "第2串"=0.0, "第3串"=0.0, "第4串"=0.0, "第5串"=0.0, "第6串"=0.0, "第7串"=0.0, "第8串"=0.0, "第9串"=0.0, "第10串"=0.0, "第11串"=0.0, "第12串"=0.0} ("1 102")
            w508 = 0.0 ("总电压")
            w509 = "" ("协议是否公开")
            n226 = local write "硬件故障"(string[][] [] ("电池故障 2")) -> ()
            n227 = local write "总电压(V)"(w508) -> ()
            n228 = local write "总电流(A)"(w508) -> ()
            n229 = local write "外总压(V)"(w508) -> ()
            n230 = local write "平均电流(A)"(w508) -> ()
            n231 = local write "SOH"(w508) -> ()
            n232 = local write "波特率"(w509) -> ()
            n233 = local write "滑动杆"(w508) -> ()
            n234 = local write "应用类型"(w509) -> ()
            n235 = local write "协议版本号"(w509) -> ()
            n236 = local write "协议是否公开"(w509) -> ()
            n237 = local write "电池充满标志位"(w509) -> ()
            n238 = local write "电池运行状态"(w509) -> ()
            n239 = local write "从板参数"(T12 {0.0, 0.0, 0.0, 0.0, 0.0, 0.0, 0.0, 0.0, 0.0, 0.0, 0.0, 0.0, 0.0, 0.0, "故障信息"="00", 0.0, 0.0, 0.0, 0.0, "RL1_ST"="", "RL2_ST"="", "RL3_ST"="", "RL4_ST"="", "RL5_ST"="", "RL6_ST"="", "RL7_ST"="", "RL8_ST"=""} ("从板参数")) -> ()
            n240 = local write "内部EE存储器状态"(w504) -> ()
            n241 = local write "系统时钟状态"(w504) -> ()
            n242 = local write "外部EE存储器状态"(w504) -> ()
            n243 = local write "供电电源状态"(w504) -> ()
            n244 = local write "温度模块检测状态"(w504) -> ()
            n245 = local write "电压模块检测状态"(w504) -> ()
            n246 = local write "绝缘检测模块状态"(w504) -> ()
            n247 = local write "电流模块模块状态"(w504) -> ()
            n248 = local write "内部总电压检测模块状态"(w504) -> ()
            n249 = local write "外部总电压检测模块状态"(w504) -> ()
            n250 = local write "电池放电均衡模块状态"(w504) -> ()
            n251 = local write "电池充电均衡模块状态"(w504) -> ()
            n252 = local write "1 102"(w506) -> ()
            n253 = local write "1"(w506) -> ()
            n254 = local write "2"(w506) -> ()
            n255 = local write "3"(w506) -> ()
            n256 = local write "4"(w506) -> ()
            n257 = local write "5"(w506) -> ()
            n258 = local write "Flash存储器状态"(w504) -> ()
            n259 = local write "1 3"(w506) -> ()
            n260 = local write "1 4"(w506) -> ()
            n261 = local write "1 6"(w506) -> ()
            n262 = local write "1 7"(w506) -> ()
          }
        }
      }
      event "刷新": Value Change {
        n263 = event-data() -> ("NewVal"=w510:bool)  [unwired: 6 out]
        n264 = case shown="真" w510 {
          frame False {
          }
          frame True {
            w512 = 0
            w514 = T9 {"第1串"=0.0, "第2串"=0.0, "第3串"=0.0, "第4串"=0.0, "第5串"=0.0, "第6串"=0.0, "第7串"=0.0, "第8串"=0.0, "第9串"=0.0, "第10串"=0.0, "第11串"=0.0, "第12串"=0.0} ("1 102")
            w516 = 0.0 ("总电压")
            w517 = "" ("协议是否公开")
            n265 = local write "硬件故障"(string[][] [] ("电池故障 2")) -> ()
            n266 = local write "总电压(V)"(w516) -> ()
            n267 = local write "总电流(A)"(w516) -> ()
            n268 = local write "外总压(V)"(w516) -> ()
            n269 = local write "平均电流(A)"(w516) -> ()
            n270 = local write "SOH"(w516) -> ()
            n271 = local write "波特率"(w517) -> ()
            n272 = local write "滑动杆"(w516) -> ()
            n273 = local write "应用类型"(w517) -> ()
            n274 = local write "协议版本号"(w517) -> ()
            n275 = local write "协议是否公开"(w517) -> ()
            n276 = local write "电池充满标志位"(w517) -> ()
            n277 = local write "电池运行状态"(w517) -> ()
            n278 = local write "从板参数"(T12 {0.0, 0.0, 0.0, 0.0, 0.0, 0.0, 0.0, 0.0, 0.0, 0.0, 0.0, 0.0, 0.0, 0.0, "故障信息"="00", 0.0, 0.0, 0.0, 0.0, "RL1_ST"="", "RL2_ST"="", "RL3_ST"="", "RL4_ST"="", "RL5_ST"="", "RL6_ST"="", "RL7_ST"="", "RL8_ST"=""} ("从板参数")) -> ()
            n279 = local write "内部EE存储器状态"(w512) -> ()
            n280 = local write "系统时钟状态"(w512) -> ()
            n281 = local write "外部EE存储器状态"(w512) -> ()
            n282 = local write "供电电源状态"(w512) -> ()
            n283 = local write "温度模块检测状态"(w512) -> ()
            n284 = local write "电压模块检测状态"(w512) -> ()
            n285 = local write "绝缘检测模块状态"(w512) -> ()
            n286 = local write "电流模块模块状态"(w512) -> ()
            n287 = local write "内部总电压检测模块状态"(w512) -> ()
            n288 = local write "外部总电压检测模块状态"(w512) -> ()
            n289 = local write "电池放电均衡模块状态"(w512) -> ()
            n290 = local write "电池充电均衡模块状态"(w512) -> ()
            n291 = local write "1 102"(w514) -> ()
            n292 = local write "1"(w514) -> ()
            n293 = local write "2"(w514) -> ()
            n294 = local write "3"(w514) -> ()
            n295 = local write "4"(w514) -> ()
            n296 = local write "5"(w514) -> ()
            n297 = local write "Flash存储器状态"(w512) -> ()
            n298 = local write "1 3"(w514) -> ()
            n299 = local write "1 4"(w514) -> ()
            n300 = local write "1 6"(w514) -> ()
            n301 = local write "1 7"(w514) -> ()
          }
        }
      }
      event Panel Close? {
        w519 = TRUE ("停止")
        n302 = event-data() -> ()  [unwired: 5 out]
        n303 = property class="VI"("FP.State"=T13."Hidden" ("前面板窗口:状态")) -> (reference out=w521:refnum<vi>, error out=w520:errorcluster)  [unwired: 2 in]
        n304 = local write "停止"(w519) -> ()
        n305 = property class="VI"(reference=w521, error in=w520, "Front Panel.Open"=FALSE ("前面板窗口:打开")) -> ()  [unwired: 2 out]
        n306 = event-data("Discard?"=w519) -> ()  [unwired: 1 in, 1 out]
      }
    }
    n307 = local write "状态"(FALSE ("状态")) -> ()
  }
  n308 = global read "功能码全局.vi" "14"() -> (w4:bool[])
  n309 = Index Array(array=w4, index=7 ("索引")) -> (element=w2:bool)
  n310 = property on="协议版本号" class="Str"("Visible"=w2) -> ()  [unwired: 2 in, 2 out]
  n311 = property on="波特率" class="Str"("Visible"=w2) -> ()  [unwired: 2 in, 2 out]
  n312 = property on="应用类型" class="Str"("Visible"=w2) -> ()  [unwired: 2 in, 2 out]
  n313 = property on="协议是否公开" class="Str"("Visible"=w2) -> ()  [unwired: 2 in, 2 out]
  n314 = call "自适应屏幕分辨率.vi"() -> ()  [unwired: 16 in]
  n315 = local write "停止"(FALSE ("停止")) -> ()
  n316 = disable-structure shown="禁用" {
    frame Disabled {
      n317 = global read "中英文全局.vi" "中英文选择"() -> (w568:enum32{"中文", "English"})
      n318 = case shown="\"中文\", 默认" w568 {
        tunnel: ["总电压(V)" "SumV(V)"] -> w567
        tunnel: ["总电流(A)" "SumCurr(A)"] -> w566
        tunnel: ["外总压(V)" "SumV_Out(V)"] -> w565
        tunnel: ["平均电流(A)" "Aver_Curr(A)"] -> w564
        tunnel: ["协议版本号" "Protocol_Ver"] -> w563
        tunnel: ["波特率" "Baudrate"] -> w562
        tunnel: ["应用类型" "Application_Type"] -> w561
        tunnel: ["协议是否公开" "Protocol_Open"] -> w560
        tunnel: ["电池运行状态" "Bat_running state"] -> w559
        tunnel: ["电池充满标志位" "Bat_full_flag"] -> w558
        tunnel: ["最高电压" "Max_V"] -> w557
        tunnel: ["位置" w662] -> w556
        tunnel: ["最低电压" "Min_V"] -> w555
        tunnel: ["位置" w662] -> w554
        tunnel: ["最高温度" "Max_T"] -> w553
        tunnel: ["位置" w662] -> w552
        tunnel: ["最低温度" "Min_T"] -> w551
        tunnel: ["位置" w662] -> w550
        tunnel: ["温差" "Diff_T"] -> w549
        tunnel: ["压差" "Diff_V"] -> w548
        tunnel: ["最高内阻" "Max_R"] -> w547
        tunnel: ["位置" w662] -> w546
        tunnel: ["最低内阻" "Min_R"] -> w545
        tunnel: ["位置" w662] -> w544
        tunnel: ["故障信息" "Fault_Info"] -> w543
        tunnel: ["最大充电总电压" "Max_Chg_SumV"] -> w542
        tunnel: ["最大充电电流" "Max_Chg_Curr"] -> w541
        tunnel: ["充电总安时" "Total_In_Ah"] -> w540
        tunnel: ["从板监控" "Slave_Monitor"] -> w539
        tunnel: ["硬件故障" "HD_Fault"] -> w538
        tunnel: ["单体电压温度" "Cellv/Temp"] -> w537
        tunnel: ["刷新" "Refresh"] -> w536
        tunnel: ["从板板号" "Slave_No."] -> w535
        tunnel: ["硬件故障" "HD_Fault"] -> w534
        tunnel: ["单板信息" "Single board information"] -> w532
        tunnel: ["串" ""] -> w530
        tunnel: ["第" ""] -> w529
        tunnel: ["电压基准" "V_reference"] -> w527
        tunnel: ["偏差" "Offset"] -> w524
        tunnel: ["温度基准" "T_reference"] -> w526
        tunnel: ["判定" "Judge"] -> w525
        frame "中文", Default {
        }
        frame "English" {
          w662 = "NO."
        }
      }
      n319 = control-ref of="本VI"() -> (w533:refnum<vi>)
      n320 = property on="总电压(V)" class="DigNum (严格)"("Caption.Text"=w567) -> ()  [unwired: 2 in, 2 out]
      n321 = property on="总电流(A)" class="DigNum (严格)"("Caption.Text"=w566) -> ()  [unwired: 2 in, 2 out]
      n322 = property on="外总压(V)" class="DigNum (严格)"("Caption.Text"=w565) -> ()  [unwired: 2 in, 2 out]
      n323 = property on="平均电流(A)" class="DigNum (严格)"("Caption.Text"=w564) -> ()  [unwired: 2 in, 2 out]
      n324 = property on="协议版本号" class="Str"("Caption.Text"=w563) -> ()  [unwired: 2 in, 2 out]
      n325 = property on="波特率" class="Str"("Caption.Text"=w562) -> ()  [unwired: 2 in, 2 out]
      n326 = property on="应用类型" class="Str"("Caption.Text"=w561) -> ()  [unwired: 2 in, 2 out]
      n327 = property on="协议是否公开" class="Str"("Caption.Text"=w560) -> ()  [unwired: 2 in, 2 out]
      n328 = property on="电池运行状态" class="Str"("Caption.Text"=w559) -> ()  [unwired: 2 in, 2 out]
      n329 = property on="电池充满标志位" class="Str"("Caption.Text"=w558) -> ()  [unwired: 2 in, 2 out]
      n330 = property on="最高电压" class="DigNum (严格)"("Caption.Text"=w557) -> ()  [unwired: 2 in, 2 out]
      n331 = property on="位置1" class="DigNum (严格)"("Caption.Text"=w556) -> ()  [unwired: 2 in, 2 out]
      n332 = property on="最低电压" class="DigNum (严格)"("Caption.Text"=w555) -> ()  [unwired: 2 in, 2 out]
      n333 = property on="位置2" class="DigNum (严格)"("Caption.Text"=w554) -> ()  [unwired: 2 in, 2 out]
      n334 = property on="最高温度" class="DigNum (严格)"("Caption.Text"=w553) -> ()  [unwired: 2 in, 2 out]
      n335 = property on="位置3" class="DigNum (严格)"("Caption.Text"=w552) -> ()  [unwired: 2 in, 2 out]
      n336 = property on="最低温度" class="DigNum (严格)"("Caption.Text"=w551) -> ()  [unwired: 2 in, 2 out]
      n337 = property on="位置4" class="DigNum (严格)"("Caption.Text"=w550) -> ()  [unwired: 2 in, 2 out]
      n338 = property on="压差" class="DigNum (严格)"("Caption.Text"=w548) -> ()  [unwired: 2 in, 2 out]
      n339 = property on="温差" class="DigNum (严格)"("Caption.Text"=w549) -> ()  [unwired: 2 in, 2 out]
      n340 = property on="最高内阻" class="DigNum (严格)"("Caption.Text"=w547) -> ()  [unwired: 2 in, 2 out]
      n341 = property on="位置5" class="DigNum (严格)"("Caption.Text"=w546) -> ()  [unwired: 2 in, 2 out]
      n342 = property on="最低内阻" class="DigNum (严格)"("Caption.Text"=w545) -> ()  [unwired: 2 in, 2 out]
      n343 = property on="位置6" class="DigNum (严格)"("Caption.Text"=w544) -> ()  [unwired: 2 in, 2 out]
      n344 = property on="故障信息" class="Str"("Caption.Text"=w543) -> ()  [unwired: 2 in, 2 out]
      n345 = property on="最大充电总电压" class="DigNum (严格)"("Caption.Text"=w542) -> ()  [unwired: 2 in, 2 out]
      n346 = property on="最大充电电流" class="DigNum (严格)"("Caption.Text"=w541) -> ()  [unwired: 2 in, 2 out]
      n347 = property on="充电总安时" class="DigNum (严格)"("Caption.Text"=w540) -> ()  [unwired: 2 in, 2 out]
      n348 = property on="单选选项2" class="Bool (严格)"("BoolText.Text"=w538) -> ()  [unwired: 2 in, 2 out]
      n349 = property on="单选选项1" class="Bool (严格)"("BoolText.Text"=w539) -> ()  [unwired: 2 in, 2 out]
      n350 = property on="单选选项2 2" class="Bool (严格)"("BoolText.Text"=w537) -> ()  [unwired: 2 in, 2 out]
      n351 = property on="刷新" class="Bool (严格)"("BoolText.Text"=w536) -> ()  [unwired: 2 in, 2 out]
      n352 = property on="电压基准" class="DigNum (严格)"("Caption.Text"=w527) -> ()  [unwired: 2 in, 2 out]
      n353 = property on="布尔" class="Bool (严格)"("Caption.Text"=w525) -> ()  [unwired: 2 in, 2 out]
      n354 = property on="布尔 2" class="Bool (严格)"("Caption.Text"=w525) -> ()  [unwired: 2 in, 2 out]
      n355 = property class="VI"(reference=w533, "Front Panel.Title"=w532) -> ()  [unwired: 1 in, 2 out]
      n356 = property on="偏差 2" class="DigNum (严格)"("Caption.Text"=w524) -> ()  [unwired: 2 in, 2 out]
      n357 = property on="偏差" class="DigNum (严格)"("Caption.Text"=w524) -> ()  [unwired: 2 in, 2 out]
      n358 = property on="从板板号 2" class="DigNum (严格)"("Caption.Text"=w535) -> ()  [unwired: 2 in, 2 out]
      n359 = property on="温度基准" class="DigNum (严格)"("Caption.Text"=w526) -> ()  [unwired: 2 in, 2 out]
      n360 = property on="硬件故障" class="Arr (严格)"("Caption.Text"=w534) -> ()  [unwired: 2 in, 2 out]
      n361 = for {
        N: 5 -> [_]
        tunnel: w530 -> [w598]
        tunnel: w529 -> [w597]
        i -> [w596]
        w599 = 12
        n362 = for {
          N: w599 -> [_]
          tunnel: [w615] -> w593 mode=indexing
          tunnel: w596 -> [w612]
          tunnel: w599 -> [w611]
          tunnel: w597 -> [w608]
          tunnel: w598 -> [w607]
          i -> [w614]
          n363 = Multiply(x=w612, y=w611) -> (x*y=w613:i32)
          n364 = Compound Arithmetic op=ADD(w614, w613, 1 ("值")) -> (w609:i32)
          n365 = Number To Decimal String(number=w609) -> (decimal integer string=w616:string)  [unwired: 1 in]
          n366 = Concatenate Strings(w608, w616, w607) -> (w615:string)
        }
        n367 = case shown="4" w596 {
          tunnel: [w602 w603 w604 w605 w606] -> w595
          frame 0, Default {
            n368 = control-ref of="1 102"() -> (w602:refnum<vi>)
          }
          frame 1 {
            n369 = control-ref of="1 3"() -> (w603:refnum<vi>)
          }
          frame 2 {
            n370 = control-ref of="1 4"() -> (w604:refnum<vi>)
          }
          frame 3 {
            n371 = control-ref of="1 6"() -> (w605:refnum<vi>)
          }
          frame 4 {
            n372 = control-ref of="1 7"() -> (w606:refnum<vi>)
          }
        }
        n373 = property class="Clust (严格)"(reference=w595) -> ("Controls[]"=w594:refnum<vi>[])  [unwired: 1 in, 2 out]
        n374 = for {
          tunnel: w594 -> [w601] mode=indexing
          tunnel: w593 -> [w600] mode=indexing
          n375 = property class="Ctl"(reference=w601, "Caption.Text"=w600) -> ()  [unwired: 1 in, 2 out]
        }
      }
      n376 = for {
        N: 5 -> [_]
        tunnel: w530 -> [w574]
        tunnel: w529 -> [w573]
        i -> [w572]
        w575 = 12
        n377 = for {
          N: w575 -> [_]
          tunnel: [w591] -> w569 mode=indexing
          tunnel: w572 -> [w588]
          tunnel: w575 -> [w587]
          tunnel: w573 -> [w584]
          tunnel: w574 -> [w583]
          i -> [w590]
          n378 = Multiply(x=w588, y=w587) -> (x*y=w589:i32)
          n379 = Compound Arithmetic op=ADD(w590, w589, 1 ("值")) -> (w585:i32)
          n380 = Number To Decimal String(number=w585) -> (decimal integer string=w592:string)  [unwired: 1 in]
          n381 = Concatenate Strings(w584, w592, w583) -> (w591:string)
        }
        n382 = case shown="4" w572 {
          tunnel: [w578 w579 w580 w581 w582] -> w571
          frame 0, Default {
            n383 = control-ref of="1"() -> (w578:refnum<vi>)
          }
          frame 1 {
            n384 = control-ref of="2"() -> (w579:refnum<vi>)
          }
          frame 2 {
            n385 = control-ref of="3"() -> (w580:refnum<vi>)
          }
          frame 3 {
            n386 = control-ref of="4"() -> (w581:refnum<vi>)
          }
          frame 4 {
            n387 = control-ref of="5"() -> (w582:refnum<vi>)
          }
        }
        n388 = property class="Clust (严格)"(reference=w571) -> ("Controls[]"=w570:refnum<vi>[])  [unwired: 1 in, 2 out]
        n389 = for {
          tunnel: w570 -> [w577] mode=indexing
          tunnel: w569 -> [w576] mode=indexing
          n390 = property class="Ctl"(reference=w577, "Caption.Text"=w576) -> ()  [unwired: 1 in, 2 out]
        }
      }
    }
    frame Enabled {
    }
  }
  n391 = while {
    stop <- w697 stop-if-true
    n392 = local read "从板板号 2"() -> (w696:u8)
    n393 = local read "布尔 2"() -> (w694:bool)
    n394 = local read "布尔"() -> (w695:bool)
    n395 = case shown="假" w694 {
      tunnel: w696 -> [_ w746]
      frame False {
        n396 = local read "布尔 3"() -> (w699:bool)
        n397 = case shown="真" w699 {
          frame False {
          }
          frame True {
            n398 = for {
              N: 5 -> [_]
              tunnel: bool[] [FALSE, FALSE, FALSE, FALSE, FALSE, FALSE, FALSE, FALSE, FALSE, FALSE, FALSE, FALSE, FALSE, FALSE, FALSE, FALSE, FALSE, FALSE, FALSE, FALSE, FALSE, FALSE, FALSE, FALSE, FALSE, FALSE, FALSE, FALSE, FALSE, FALSE, FALSE, FALSE, FALSE, FALSE, FALSE, FALSE, FALSE, FALSE, FALSE, FALSE, FALSE, FALSE, FALSE, FALSE, FALSE, FALSE, FALSE, FALSE, FALSE, FALSE, FALSE, FALSE, FALSE, FALSE, FALSE, FALSE, FALSE, FALSE, FALSE, FALSE] -> [w705]
              i -> [w704]
              w706 = 12 ("y")
              n399 = Multiply(x=w704, y=w706) -> (x*y=w707:i32)
              n400 = Array Subset(array=w705, index=w707, length=w706) -> (w703:bool[])
              n401 = case shown="4" w704 {
                tunnel: w703 -> [w709 w716 w723 w730 w737]
                frame 0, Default {
                  n402 = control-ref of="1"() -> (w708:refnum<vi>)
                  n403 = property class="Clust (严格)"(reference=w708) -> ("Controls[]"=w710:refnum<vi>[])  [unwired: 1 in, 2 out]
                  n404 = for {
                    tunnel: w710 -> [w713] mode=indexing
                    tunnel: w709 -> [w714]
                    i -> [w711]
                    n405 = Index Array(array=w714, index=w711) -> (element=w712:bool)
                    n406 = property class="Ctl"(reference=w713, "Blinking"=w712) -> ()  [unwired: 1 in, 2 out]
                  }
                }
                frame 1 {
                  n407 = control-ref of="2"() -> (w715:refnum<vi>)
                  n408 = property class="Clust (严格)"(reference=w715) -> ("Controls[]"=w717:refnum<vi>[])  [unwired: 1 in, 2 out]
                  n409 = for {
                    tunnel: w717 -> [w720] mode=indexing
                    tunnel: w716 -> [w721]
                    i -> [w718]
                    n410 = Index Array(array=w721, index=w718) -> (element=w719:bool)
                    n411 = property class="Ctl"(reference=w720, "Blinking"=w719) -> ()  [unwired: 1 in, 2 out]
                  }
                }
                frame 2 {
                  n412 = control-ref of="3"() -> (w722:refnum<vi>)
                  n413 = property class="Clust (严格)"(reference=w722) -> ("Controls[]"=w724:refnum<vi>[])  [unwired: 1 in, 2 out]
                  n414 = for {
                    tunnel: w724 -> [w727] mode=indexing
                    tunnel: w723 -> [w728]
                    i -> [w725]
                    n415 = Index Array(array=w728, index=w725) -> (element=w726:bool)
                    n416 = property class="Ctl"(reference=w727, "Blinking"=w726) -> ()  [unwired: 1 in, 2 out]
                  }
                }
                frame 3 {
                  n417 = control-ref of="4"() -> (w729:refnum<vi>)
                  n418 = property class="Clust (严格)"(reference=w729) -> ("Controls[]"=w731:refnum<vi>[])  [unwired: 1 in, 2 out]
                  n419 = for {
                    tunnel: w731 -> [w734] mode=indexing
                    tunnel: w730 -> [w735]
                    i -> [w732]
                    n420 = Index Array(array=w735, index=w732) -> (element=w733:bool)
                    n421 = property class="Ctl"(reference=w734, "Blinking"=w733) -> ()  [unwired: 1 in, 2 out]
                  }
                }
                frame 4 {
                  n422 = control-ref of="5"() -> (w736:refnum<vi>)
                  n423 = property class="Clust (严格)"(reference=w736) -> ("Controls[]"=w738:refnum<vi>[])  [unwired: 1 in, 2 out]
                  n424 = for {
                    tunnel: w738 -> [w741] mode=indexing
                    tunnel: w737 -> [w742]
                    i -> [w739]
                    n425 = Index Array(array=w742, index=w739) -> (element=w740:bool)
                    n426 = property class="Ctl"(reference=w741, "Blinking"=w740) -> ()  [unwired: 1 in, 2 out]
                  }
                }
              }
            }
            n427 = local write "布尔 3"(FALSE ("布尔 3")) -> ()
          }
        }
      }
      frame True {
        n428 = global read "单体信息全局.vi" "位置 2"() -> (w747:i32[])
        n429 = while {
          tunnel: w747 -> [w809]
          tunnel: w746 -> [w808]
          shift-right: [w805] -> _
          shift-left: 0 ("index of element") -> [w804]
          tunnel: [w803] -> w751 mode=indexing
          tunnel: [w802] -> w750
          i -> [w802]
          stop <- w806 stop-if-true
          n430 = Search 1D Array(1D array=w809, element=w808, start index (0)=w804) -> (index of element=w803:i32)
          n431 = Equal?(x=w803, y=-1) -> (x = y?=w806:bool)
          n432 = Increment(x=w803) -> (x+1=w805:i32)
        }
        n433 = global read "单体信息全局.vi" "数据 2"() -> (w749:dbl[])
        n434 = Reshape Array(w751, w750) -> (w752:i32[])
        n435 = for {
          tunnel: w749 -> [w801]
          tunnel: w752 -> [w800] mode=indexing
          tunnel: [w793] -> w744 mode=indexing
          n436 = local read "温度基准"() -> (w796:dbl)
          n437 = local read "偏差"() -> (w795:dbl)
          n438 = Index Array(array=w801, index=w800) -> (element=w797:dbl)
          n439 = Add(x=w796, y=w795) -> (x+y=w798:dbl)
          n440 = Subtract(x=w796, y=w795) -> (x-y=w799:dbl)
          n441 = In Range and Coerce(upper limit=w798, x=w797, lower limit=w799) -> (In Range?=w794:bool)  [unwired: 1 out]
          n442 = Not(x=w794) -> (.not. x?=w793:bool)
        }
        n443 = for {
          N: 5 -> [_]
          tunnel: w744 -> [w755]
          i -> [w754]
          w756 = 12 ("y")
          n444 = Multiply(x=w754, y=w756) -> (x*y=w757:i32)
          n445 = Array Subset(array=w755, index=w757, length=w756) -> (w753:bool[])
          n446 = case shown="2" w754 {
            tunnel: w753 -> [w759 w766 w773 w780 w787]
            frame 0, Default {
              n447 = control-ref of="1"() -> (w758:refnum<vi>)
              n448 = property class="Clust (严格)"(reference=w758) -> ("Controls[]"=w760:refnum<vi>[])  [unwired: 1 in, 2 out]
              n449 = for {
                tunnel: w760 -> [w763] mode=indexing
                tunnel: w759 -> [w764]
                i -> [w761]
                n450 = Index Array(array=w764, index=w761) -> (element=w762:bool)
                n451 = property class="Ctl"(reference=w763, "Blinking"=w762) -> ()  [unwired: 1 in, 2 out]
              }
            }
            frame 1 {
              n452 = control-ref of="2"() -> (w765:refnum<vi>)
              n453 = property class="Clust (严格)"(reference=w765) -> ("Controls[]"=w767:refnum<vi>[])  [unwired: 1 in, 2 out]
              n454 = for {
                tunnel: w767 -> [w770] mode=indexing
                tunnel: w766 -> [w771]
                i -> [w768]
                n455 = Index Array(array=w771, index=w768) -> (element=w769:bool)
                n456 = property class="Ctl"(reference=w770, "Blinking"=w769) -> ()  [unwired: 1 in, 2 out]
              }
            }
            frame 2 {
              n457 = control-ref of="3"() -> (w772:refnum<vi>)
              n458 = property class="Clust (严格)"(reference=w772) -> ("Controls[]"=w774:refnum<vi>[])  [unwired: 1 in, 2 out]
              n459 = for {
                tunnel: w774 -> [w777] mode=indexing
                tunnel: w773 -> [w778]
                i -> [w775]
                n460 = Index Array(array=w778, index=w775) -> (element=w776:bool)
                n461 = property class="Ctl"(reference=w777, "Blinking"=w776) -> ()  [unwired: 1 in, 2 out]
              }
            }
            frame 3 {
              n462 = control-ref of="4"() -> (w779:refnum<vi>)
              n463 = property class="Clust (严格)"(reference=w779) -> ("Controls[]"=w781:refnum<vi>[])  [unwired: 1 in, 2 out]
              n464 = for {
                tunnel: w781 -> [w784] mode=indexing
                tunnel: w780 -> [w785]
                i -> [w782]
                n465 = Index Array(array=w785, index=w782) -> (element=w783:bool)
                n466 = property class="Ctl"(reference=w784, "Blinking"=w783) -> ()  [unwired: 1 in, 2 out]
              }
            }
            frame 4 {
              n467 = control-ref of="5"() -> (w786:refnum<vi>)
              n468 = property class="Clust (严格)"(reference=w786) -> ("Controls[]"=w788:refnum<vi>[])  [unwired: 1 in, 2 out]
              n469 = for {
                tunnel: w788 -> [w791] mode=indexing
                tunnel: w787 -> [w792]
                i -> [w789]
                n470 = Index Array(array=w792, index=w789) -> (element=w790:bool)
                n471 = property class="Ctl"(reference=w791, "Blinking"=w790) -> ()  [unwired: 1 in, 2 out]
              }
            }
          }
        }
        n472 = local write "布尔 3"(TRUE ("布尔 3")) -> ()
      }
    }
    n473 = case shown="假" w695 {
      tunnel: w696 -> [_ w857]
      frame False {
        n474 = local read "布尔 3"() -> (w810:bool)
        n475 = case shown="真" w810 {
          frame False {
          }
          frame True {
            n476 = local write "布尔 3"(FALSE ("布尔 3")) -> ()
            n477 = for {
              N: 5 -> [_]
              tunnel: bool[] [FALSE, FALSE, FALSE, FALSE, FALSE, FALSE, FALSE, FALSE, FALSE, FALSE, FALSE, FALSE, FALSE, FALSE, FALSE, FALSE, FALSE, FALSE, FALSE, FALSE, FALSE, FALSE, FALSE, FALSE, FALSE, FALSE, FALSE, FALSE, FALSE, FALSE, FALSE, FALSE, FALSE, FALSE, FALSE, FALSE, FALSE, FALSE, FALSE, FALSE, FALSE, FALSE, FALSE, FALSE, FALSE, FALSE, FALSE, FALSE, FALSE, FALSE, FALSE, FALSE, FALSE, FALSE, FALSE, FALSE, FALSE, FALSE, FALSE, FALSE] -> [w816]
              i -> [w815]
              w817 = 12 ("y")
              n478 = Multiply(x=w815, y=w817) -> (x*y=w818:i32)
              n479 = Array Subset(array=w816, index=w818, length=w817) -> (w814:bool[])
              n480 = case shown="0, 默认" w815 {
                tunnel: w814 -> [w820 w827 w834 w841 w848]
                frame 0, Default {
                  n481 = control-ref of="1 102"() -> (w819:refnum<vi>)
                  n482 = property class="Clust (严格)"(reference=w819) -> ("Controls[]"=w821:refnum<vi>[])  [unwired: 1 in, 2 out]
                  n483 = for {
                    tunnel: w821 -> [w825] mode=indexing
                    tunnel: w820 -> [w824]
                    i -> [w823]
                    n484 = Index Array(array=w824, index=w823) -> (element=w822:bool)
                    n485 = property class="Ctl"(reference=w825, "Blinking"=w822) -> ()  [unwired: 1 in, 2 out]
                  }
                }
                frame 1 {
                  n486 = control-ref of="1 3"() -> (w826:refnum<vi>)
                  n487 = property class="Clust (严格)"(reference=w826) -> ("Controls[]"=w828:refnum<vi>[])  [unwired: 1 in, 2 out]
                  n488 = for {
                    tunnel: w828 -> [w831] mode=indexing
                    tunnel: w827 -> [w832]
                    i -> [w829]
                    n489 = Index Array(array=w832, index=w829) -> (element=w830:bool)
                    n490 = property class="Ctl"(reference=w831, "Blinking"=w830) -> ()  [unwired: 1 in, 2 out]
                  }
                }
                frame 2 {
                  n491 = control-ref of="1 4"() -> (w833:refnum<vi>)
                  n492 = property class="Clust (严格)"(reference=w833) -> ("Controls[]"=w835:refnum<vi>[])  [unwired: 1 in, 2 out]
                  n493 = for {
                    tunnel: w835 -> [w838] mode=indexing
                    tunnel: w834 -> [w839]
                    i -> [w836]
                    n494 = Index Array(array=w839, index=w836) -> (element=w837:bool)
                    n495 = property class="Ctl"(reference=w838, "Blinking"=w837) -> ()  [unwired: 1 in, 2 out]
                  }
                }
                frame 3 {
                  n496 = control-ref of="1 6"() -> (w840:refnum<vi>)
                  n497 = property class="Clust (严格)"(reference=w840) -> ("Controls[]"=w842:refnum<vi>[])  [unwired: 1 in, 2 out]
                  n498 = for {
                    tunnel: w842 -> [w845] mode=indexing
                    tunnel: w841 -> [w846]
                    i -> [w843]
                    n499 = Index Array(array=w846, index=w843) -> (element=w844:bool)
                    n500 = property class="Ctl"(reference=w845, "Blinking"=w844) -> ()  [unwired: 1 in, 2 out]
                  }
                }
                frame 4 {
                  n501 = control-ref of="1 7"() -> (w847:refnum<vi>)
                  n502 = property class="Clust (严格)"(reference=w847) -> ("Controls[]"=w849:refnum<vi>[])  [unwired: 1 in, 2 out]
                  n503 = for {
                    tunnel: w849 -> [w852] mode=indexing
                    tunnel: w848 -> [w853]
                    i -> [w850]
                    n504 = Index Array(array=w853, index=w850) -> (element=w851:bool)
                    n505 = property class="Ctl"(reference=w852, "Blinking"=w851) -> ()  [unwired: 1 in, 2 out]
                  }
                }
              }
            }
          }
        }
      }
      frame True {
        n506 = global read "单体信息全局.vi" "位置"() -> (w863:i32[])
        n507 = while {
          tunnel: w863 -> [w920]
          tunnel: w857 -> [w919]
          shift-right: [w916] -> _
          shift-left: 0 ("index of element") -> [w915]
          tunnel: [w914] -> w859 mode=indexing
          tunnel: [w913] -> w860
          i -> [w913]
          stop <- w917 stop-if-true
          n508 = Search 1D Array(1D array=w920, element=w919, start index (0)=w915) -> (index of element=w914:i32)
          n509 = Equal?(x=w914, y=-1) -> (x = y?=w917:bool)
          n510 = Increment(x=w914) -> (x+1=w916:i32)
        }
        n511 = global read "单体信息全局.vi" "数据"() -> (w861:dbl[])
        n512 = Reshape Array(w859, w860) -> (w858:i32[])
        n513 = for {
          tunnel: w861 -> [w912]
          tunnel: w858 -> [w911] mode=indexing
          tunnel: [w904] -> w855 mode=indexing
          n514 = local read "电压基准"() -> (w909:dbl)
          n515 = local read "偏差 2"() -> (w908:dbl)
          n516 = Index Array(array=w912, index=w911) -> (element=w910:dbl)
          n517 = Add(x=w909, y=w908) -> (x+y=w907:dbl)
          n518 = Subtract(x=w909, y=w908) -> (x-y=w906:dbl)
          n519 = In Range and Coerce(upper limit=w907, x=w910, lower limit=w906) -> (In Range?=w905:bool)  [unwired: 1 out]
          n520 = Not(x=w905) -> (.not. x?=w904:bool)
        }
        n521 = local write "布尔 3"(TRUE ("布尔 3")) -> ()
        n522 = for {
          N: 5 -> [_]
          tunnel: w855 -> [w866]
          i -> [w865]
          w867 = 12 ("y")
          n523 = Multiply(x=w865, y=w867) -> (x*y=w868:i32)
          n524 = Array Subset(array=w866, index=w868, length=w867) -> (w864:bool[])
          n525 = case shown="1" w865 {
            tunnel: w864 -> [w870 w877 w884 w891 w898]
            frame 0, Default {
              n526 = control-ref of="1 102"() -> (w869:refnum<vi>)
              n527 = property class="Clust (严格)"(reference=w869) -> ("Controls[]"=w871:refnum<vi>[])  [unwired: 1 in, 2 out]
              n528 = for {
                tunnel: w871 -> [w875] mode=indexing
                tunnel: w870 -> [w874]
                i -> [w873]
                n529 = Index Array(array=w874, index=w873) -> (element=w872:bool)
                n530 = property class="Ctl"(reference=w875, "Blinking"=w872) -> ()  [unwired: 1 in, 2 out]
              }
            }
            frame 1 {
              n531 = control-ref of="1 3"() -> (w876:refnum<vi>)
              n532 = property class="Clust (严格)"(reference=w876) -> ("Controls[]"=w878:refnum<vi>[])  [unwired: 1 in, 2 out]
              n533 = for {
                tunnel: w878 -> [w881] mode=indexing
                tunnel: w877 -> [w882]
                i -> [w879]
                n534 = Index Array(array=w882, index=w879) -> (element=w880:bool)
                n535 = property class="Ctl"(reference=w881, "Blinking"=w880) -> ()  [unwired: 1 in, 2 out]
              }
            }
            frame 2 {
              n536 = control-ref of="1 4"() -> (w883:refnum<vi>)
              n537 = property class="Clust (严格)"(reference=w883) -> ("Controls[]"=w885:refnum<vi>[])  [unwired: 1 in, 2 out]
              n538 = for {
                tunnel: w885 -> [w888] mode=indexing
                tunnel: w884 -> [w889]
                i -> [w886]
                n539 = Index Array(array=w889, index=w886) -> (element=w887:bool)
                n540 = property class="Ctl"(reference=w888, "Blinking"=w887) -> ()  [unwired: 1 in, 2 out]
              }
            }
            frame 3 {
              n541 = control-ref of="1 6"() -> (w890:refnum<vi>)
              n542 = property class="Clust (严格)"(reference=w890) -> ("Controls[]"=w892:refnum<vi>[])  [unwired: 1 in, 2 out]
              n543 = for {
                tunnel: w892 -> [w895] mode=indexing
                tunnel: w891 -> [w896]
                i -> [w893]
                n544 = Index Array(array=w896, index=w893) -> (element=w894:bool)
                n545 = property class="Ctl"(reference=w895, "Blinking"=w894) -> ()  [unwired: 1 in, 2 out]
              }
            }
            frame 4 {
              n546 = control-ref of="1 7"() -> (w897:refnum<vi>)
              n547 = property class="Clust (严格)"(reference=w897) -> ("Controls[]"=w899:refnum<vi>[])  [unwired: 1 in, 2 out]
              n548 = for {
                tunnel: w899 -> [w902] mode=indexing
                tunnel: w898 -> [w903]
                i -> [w900]
                n549 = Index Array(array=w903, index=w900) -> (element=w901:bool)
                n550 = property class="Ctl"(reference=w902, "Blinking"=w901) -> ()  [unwired: 1 in, 2 out]
              }
            }
          }
        }
      }
    }
    n551 = Wait Until Next ms Multiple(millisecond multiple=u32 1000 ("毫秒倍数")) -> ()  [unwired: 1 out]
    n552 = local read "停止"() -> (w697:bool)
  }
  n553 = while {
    stop <- w922 stop-if-true
    n554 = local read "选项卡控件"() -> (w921:enum32{"从板监控", "从板信息2", "电压温度", "高压板监控"})
    n555 = case shown="\"电压温度\"" w921 {
      frame "从板监控", Default {
      }
      frame "电压温度" {
        n556 = local read "从板板号 2"() -> (w925:u8)
        n557 = global read "单体信息全局.vi" "温度数据"() -> (w926:u8[][])
        n558 = global read "从板全局变量.vi" "温度个数"() -> (w929:u8[])
        n559 = Decrement(x=w925) -> (x-1=w927:u8)
        n560 = Decrement(x=w925) -> (x-1=w928:u8)
        n561 = global read "单体信息全局.vi" "单体数据"() -> (w938:dbl[][])
        n562 = global read "从板全局变量.vi" "电池节数"() -> (w935:u8[])
        n563 = Decrement(x=w925) -> (x-1=w937:u8)
        n564 = Decrement(x=w925) -> (x-1=w936:u8)
        n565 = Index Array(array=w926, index (row)=w927) -> (element=w930:u8[])  [unwired: 1 in]
        n566 = Index Array(array=w929, index=w928) -> (element=w931:u8)
        n567 = Index Array(array=w938, index (row)=w937) -> (element=w934:dbl[])  [unwired: 1 in]
        n568 = Index Array(array=w935, index=w936) -> (element=w933:u8)
        n569 = Array Subset(array=w930, length=w931) -> (w924:u8[])  [unwired: 1 in]
        n570 = Array Subset(array=w934, length=w933) -> (w932:dbl[])  [unwired: 1 in]
        n571 = for {
          tunnel: [w1080] -> w950 mode=indexing
          tunnel: [TRUE] -> w939 mode=indexing
          tunnel: w924 -> [w1080] mode=indexing
        }
        n572 = for {
          tunnel: [w1093] -> w951 mode=indexing
          tunnel: [TRUE] -> w941 mode=indexing
          tunnel: w932 -> [w1093] mode=indexing
        }
        n573 = Array Size(array=w950) -> (size(s)=w948:i32)
        n574 = Array Size(array=w951) -> (size(s)=w953:i32)
        n575 = Quotient & Remainder(x=w948, y=12) -> (x-y*floor(x/y)=w944:i32, floor(x/y)=w946:i32)
        n576 = for {
          N: 5 -> [_]
          tunnel: w941 -> [w1016]
          i -> [w1015]
          w1017 = 12 ("y")
          n577 = Multiply(x=w1015, y=w1017) -> (x*y=w1018:i32)
          n578 = Array Subset(array=w1016, index=w1018, length=w1017) -> (w1014:bool[])
          n579 = case shown="4" w1015 {
            tunnel: w1014 -> [w1020 w1030 w1040 w1050 w1060]
            frame 0, Default {
              n580 = control-ref of="1 102"() -> (w1019:refnum<vi>)
              n581 = property class="Clust (严格)"(reference=w1019) -> ("Controls[]"=w1021:refnum<vi>[])  [unwired: 1 in, 2 out]
              n582 = for {
                tunnel: w1021 -> [w1028] mode=indexing
                tunnel: w1020 -> [w1027]
                i -> [w1026]
                n583 = Index Array(array=w1027, index=w1026) -> (element=w1025:bool)
                n584 = Select(t=0, s=w1025, f=2) -> (s? t:f=w1022:i32)
                n585 = property class="Ctl"(reference=w1028, "DisabledEnum"=w1022) -> ()  [unwired: 1 in, 2 out]
              }
            }
            frame 1 {
              n586 = control-ref of="1 3"() -> (w1029:refnum<vi>)
              n587 = property class="Clust (严格)"(reference=w1029) -> ("Controls[]"=w1031:refnum<vi>[])  [unwired: 1 in, 2 out]
              n588 = for {
                tunnel: w1031 -> [w1037] mode=indexing
                tunnel: w1030 -> [w1038]
                i -> [w1036]
                n589 = Index Array(array=w1038, index=w1036) -> (element=w1033:bool)
                n590 = Select(t=0, s=w1033, f=2) -> (s? t:f=w1032:i32)
                n591 = property class="Ctl"(reference=w1037, "DisabledEnum"=w1032) -> ()  [unwired: 1 in, 2 out]
              }
            }
            frame 2 {
              n592 = control-ref of="1 4"() -> (w1039:refnum<vi>)
              n593 = property class="Clust (严格)"(reference=w1039) -> ("Controls[]"=w1041:refnum<vi>[])  [unwired: 1 in, 2 out]
              n594 = for {
                tunnel: w1041 -> [w1047] mode=indexing
                tunnel: w1040 -> [w1048]
                i -> [w1046]
                n595 = Index Array(array=w1048, index=w1046) -> (element=w1043:bool)
                n596 = Select(t=0, s=w1043, f=2) -> (s? t:f=w1042:i32)
                n597 = property class="Ctl"(reference=w1047, "DisabledEnum"=w1042) -> ()  [unwired: 1 in, 2 out]
              }
            }
            frame 3 {
              n598 = control-ref of="1 6"() -> (w1049:refnum<vi>)
              n599 = property class="Clust (严格)"(reference=w1049) -> ("Controls[]"=w1051:refnum<vi>[])  [unwired: 1 in, 2 out]
              n600 = for {
                tunnel: w1051 -> [w1057] mode=indexing
                tunnel: w1050 -> [w1058]
                i -> [w1056]
                n601 = Index Array(array=w1058, index=w1056) -> (element=w1053:bool)
                n602 = Select(t=0, s=w1053, f=2) -> (s? t:f=w1052:i32)
                n603 = property class="Ctl"(reference=w1057, "DisabledEnum"=w1052) -> ()  [unwired: 1 in, 2 out]
              }
            }
            frame 4 {
              n604 = control-ref of="1 7"() -> (w1059:refnum<vi>)
              n605 = property class="Clust (严格)"(reference=w1059) -> ("Controls[]"=w1061:refnum<vi>[])  [unwired: 1 in, 2 out]
              n606 = for {
                tunnel: w1061 -> [w1067] mode=indexing
                tunnel: w1060 -> [w1068]
                i -> [w1066]
                n607 = Index Array(array=w1068, index=w1066) -> (element=w1063:bool)
                n608 = Select(t=0, s=w1063, f=2) -> (s? t:f=w1062:i32)
                n609 = property class="Ctl"(reference=w1067, "DisabledEnum"=w1062) -> ()  [unwired: 1 in, 2 out]
              }
            }
          }
        }
        n610 = Quotient & Remainder(x=w953, y=12) -> (x-y*floor(x/y)=w957:i32, floor(x/y)=w955:i32)
        n611 = Equal To 0?(x=w944) -> (x = 0?=w945:bool)
        n612 = for {
          N: 5 -> [_]
          tunnel: w939 -> [w961]
          i -> [w960]
          w962 = 12 ("y")
          n613 = Multiply(x=w960, y=w962) -> (x*y=w963:i32)
          n614 = Array Subset(array=w961, index=w963, length=w962) -> (w959:bool[])
          n615 = case shown="1" w960 {
            tunnel: w959 -> [w965 w975 w985 w995 w1005]
            frame 0, Default {
              n616 = control-ref of="1"() -> (w964:refnum<vi>)
              n617 = property class="Clust (严格)"(reference=w964) -> ("Controls[]"=w966:refnum<vi>[])  [unwired: 1 in, 2 out]
              n618 = for {
                tunnel: w966 -> [w972] mode=indexing
                tunnel: w965 -> [w973]
                i -> [w971]
                n619 = Index Array(array=w973, index=w971) -> (element=w968:bool)
                n620 = Select(t=0, s=w968, f=2) -> (s? t:f=w967:i32)
                n621 = property class="Ctl"(reference=w972, "DisabledEnum"=w967) -> ()  [unwired: 1 in, 2 out]
              }
            }
            frame 1 {
              n622 = control-ref of="2"() -> (w974:refnum<vi>)
              n623 = property class="Clust (严格)"(reference=w974) -> ("Controls[]"=w976:refnum<vi>[])  [unwired: 1 in, 2 out]
              n624 = for {
                tunnel: w976 -> [w982] mode=indexing
                tunnel: w975 -> [w983]
                i -> [w981]
                n625 = Index Array(array=w983, index=w981) -> (element=w978:bool)
                n626 = Select(t=0, s=w978, f=2) -> (s? t:f=w977:i32)
                n627 = property class="Ctl"(reference=w982, "DisabledEnum"=w977) -> ()  [unwired: 1 in, 2 out]
              }
            }
            frame 2 {
              n628 = control-ref of="3"() -> (w984:refnum<vi>)
              n629 = property class="Clust (严格)"(reference=w984) -> ("Controls[]"=w986:refnum<vi>[])  [unwired: 1 in, 2 out]
              n630 = for {
                tunnel: w986 -> [w992] mode=indexing
                tunnel: w985 -> [w993]
                i -> [w991]
                n631 = Index Array(array=w993, index=w991) -> (element=w988:bool)
                n632 = Select(t=0, s=w988, f=2) -> (s? t:f=w987:i32)
                n633 = property class="Ctl"(reference=w992, "DisabledEnum"=w987) -> ()  [unwired: 1 in, 2 out]
              }
            }
            frame 3 {
              n634 = control-ref of="4"() -> (w994:refnum<vi>)
              n635 = property class="Clust (严格)"(reference=w994) -> ("Controls[]"=w996:refnum<vi>[])  [unwired: 1 in, 2 out]
              n636 = for {
                tunnel: w996 -> [w1002] mode=indexing
                tunnel: w995 -> [w1003]
                i -> [w1001]
                n637 = Index Array(array=w1003, index=w1001) -> (element=w998:bool)
                n638 = Select(t=0, s=w998, f=2) -> (s? t:f=w997:i32)
                n639 = property class="Ctl"(reference=w1002, "DisabledEnum"=w997) -> ()  [unwired: 1 in, 2 out]
              }
            }
            frame 4 {
              n640 = control-ref of="5"() -> (w1004:refnum<vi>)
              n641 = property class="Clust (严格)"(reference=w1004) -> ("Controls[]"=w1006:refnum<vi>[])  [unwired: 1 in, 2 out]
              n642 = for {
                tunnel: w1006 -> [w1012] mode=indexing
                tunnel: w1005 -> [w1013]
                i -> [w1011]
                n643 = Index Array(array=w1013, index=w1011) -> (element=w1008:bool)
                n644 = Select(t=0, s=w1008, f=2) -> (s? t:f=w1007:i32)
                n645 = property class="Ctl"(reference=w1012, "DisabledEnum"=w1007) -> ()  [unwired: 1 in, 2 out]
              }
            }
          }
        }
        n646 = Equal To 0?(x=w957) -> (x = 0?=w956:bool)
        n647 = Increment(x=w946) -> (x+1=w947:i32)
        n648 = Increment(x=w955) -> (x+1=w954:i32)
        n649 = Select(t=w955, s=w956, f=w954) -> (s? t:f=w952:i32)
        n650 = Select(t=w946, s=w945, f=w947) -> (s? t:f=w949:i32)
        n651 = for {
          N: w949 -> [_]
          tunnel: w950 -> [w1074]
          i -> [w1071]
          w1072 = 12 ("y")
          n652 = Multiply(x=w1071, y=w1072) -> (x*y=w1073:i32)
          n653 = Array Subset(array=w1074, index=w1073, length=w1072) -> (w1070:u8[])
          n654 = Array To Cluster(array=w1070) -> (cluster=w1069:T14)
          n655 = case shown="1" w1071 {
            tunnel: w1069 -> [w1075 w1076 w1077 w1078 w1079]
            frame 0, Default {
              n656 = local write "1"(w1075) -> ()
            }
            frame 1 {
              n657 = local write "2"(w1076) -> ()
            }
            frame 2 {
              n658 = local write "3"(w1077) -> ()
            }
            frame 3 {
              n659 = local write "4"(w1078) -> ()
            }
            frame 4 {
              n660 = local write "5"(w1079) -> ()
            }
          }
        }
        n661 = for {
          N: w952 -> [_]
          tunnel: w951 -> [w1087]
          i -> [w1084]
          w1085 = 12 ("y")
          n662 = Multiply(x=w1084, y=w1085) -> (x*y=w1086:i32)
          n663 = Array Subset(array=w1087, index=w1086, length=w1085) -> (w1083:dbl[])
          n664 = Array To Cluster(array=w1083) -> (cluster=w1082:T15)
          n665 = case shown="3" w1084 {
            tunnel: w1082 -> [w1088 w1089 w1090 w1091 w1092]
            frame 0, Default {
              n666 = local write "1 102"(w1088) -> ()
            }
            frame 1 {
              n667 = local write "1 3"(w1089) -> ()
            }
            frame 2 {
              n668 = local write "1 4"(w1090) -> ()
            }
            frame 3 {
              n669 = local write "1 6"(w1091) -> ()
            }
            frame 4 {
              n670 = local write "1 7"(w1092) -> ()
            }
          }
        }
      }
    }
    n671 = Wait Until Next ms Multiple(millisecond multiple=u32 500 ("毫秒倍数")) -> ()  [unwired: 1 out]
    n672 = local read "停止"() -> (w922:bool)
  }
  n673 = while {
    stop <- "停止" stop-if-true
    n674 = local read "从板板号 2"() -> (w1184:u8)
    n675 = global read "从板全局变量.vi" "最高电压位置"() -> (w1180:dbl[])
    n676 = global read "从板全局变量.vi" "最低电压位置"() -> (w1179:dbl[])
    n677 = global read "从板全局变量.vi" "最高温度位置"() -> (w1176:dbl[])
    n678 = global read "从板全局变量.vi" "最低温度位置"() -> (w1175:dbl[])
    n679 = global read "从板全局变量.vi" "最高电压"() -> (w1182:dbl[])
    n680 = global read "从板全局变量.vi" "最低电压"() -> (w1181:dbl[])
    n681 = global read "从板全局变量.vi" "最高温度"() -> (w1178:dbl[])
    n682 = global read "从板全局变量.vi" "最低温度"() -> (w1177:dbl[])
    n683 = global read "从板全局变量.vi" "总电压"() -> (w1185:dbl[])
    n684 = Decrement(x=w1184) -> (x-1=w1101:u8)
    n685 = disable-structure shown="禁用" {
      disable-tunnel: w1101 -> [w1198 _]
      frame Disabled {
        n686 = global read "从板全局变量.vi" "平均电流"() -> (w1202:dbl[])
        n687 = global read "从板全局变量.vi" "外总压"() -> (w1204:dbl[])
        n688 = global read "从板全局变量.vi" "总电流"() -> (w1201:dbl[])
        n689 = Index Array(array=w1204, index=w1198) -> (element=w1203:dbl)
        n690 = Index Array(array=w1202, index=w1198) -> (element=w1200:dbl)
        n691 = Index Array(array=w1201, index=w1198) -> (element=w1199:dbl)
        n692 = local write "外总压(V)"(w1203) -> ()
        n693 = local write "总电流(A)"(w1199) -> ()
        n694 = local write "平均电流(A)"(w1200) -> ()
      }
      frame Enabled {
      }
    }
    n695 = disable-structure shown="禁用" {
      disable-tunnel: w1101 -> [w1214 _]
      frame Disabled {
        n696 = global read "从板全局变量.vi" "SOH"() -> (w1217:dbl[])
        n697 = global read "从板全局变量.vi" "SOC"() -> (w1218:dbl[])
        n698 = Index Array(array=w1218, index=w1214) -> (element=w1216:dbl)
        n699 = Index Array(array=w1217, index=w1214) -> (element=w1215:dbl)
        n700 = local write "滑动杆"(w1216) -> ()
        n701 = local write "SOH"(w1215) -> ()
      }
      frame Enabled {
      }
    }
    n702 = Index Array(array=w1185, index=w1101) -> (element=w1183:dbl)
    n703 = Index Array(array=w1176, index=w1101) -> (element=→"最高温度位置":dbl)
    n704 = Index Array(array=w1179, index=w1101) -> (element=→"最低电压位置":dbl)
    n705 = Index Array(array=w1178, index=w1101) -> (element=→"最高温度":dbl)
    n706 = Index Array(array=w1182, index=w1101) -> (element=→"最高电压":dbl)
    n707 = Index Array(array=w1181, index=w1101) -> (element=→"最低电压":dbl)
    n708 = Index Array(array=w1177, index=w1101) -> (element=→"最低温度":dbl)
    n709 = Index Array(array=w1180, index=w1101) -> (element=→"最高电压位置":dbl)
    n710 = Index Array(array=w1175, index=w1101) -> (element=→"最低温度位置":dbl)
    n711 = local write "总电压(V)"(w1183) -> ()
    n712 = global read "从板全局变量.vi" "协议是否公开"() -> (w1161:string[])
    n713 = global read "从板全局变量.vi" "电池运行状态"() -> (w1162:string[])
    n714 = disable-structure shown="禁用" {
      disable-tunnel: w1101 -> [w1205 _]
      frame Disabled {
        n715 = global read "从板全局变量.vi" "最大内阻位置"() -> (w1212:dbl[])
        n716 = global read "从板全局变量.vi" "最小内阻位置"() -> (w1213:dbl[])
        n717 = global read "从板全局变量.vi" "最大内阻"() -> (w1210:dbl[])
        n718 = global read "从板全局变量.vi" "最小内阻"() -> (w1211:dbl[])
        n719 = Index Array(array=w1210, index=w1205) -> (element=→"最大内阻":dbl)
        n720 = Index Array(array=w1211, index=w1205) -> (element=→"最小内阻":dbl)
        n721 = Index Array(array=w1212, index=w1205) -> (element=→"最大内阻位置":dbl)
        n722 = Index Array(array=w1213, index=w1205) -> (element=→"最小内阻位置":dbl)
      }
      frame Enabled {
      }
    }
    n723 = global read "从板全局变量.vi" "故障信息"() -> (w1157:string[])
    n724 = global read "从板全局变量.vi" "应用类型"() -> (w1159:string[])
    n725 = global read "从板全局变量.vi" "继电器1"() -> (w1164:dbl[])
    n726 = global read "从板全局变量.vi" "继电器2"() -> (w1165:dbl[])
    n727 = global read "从板全局变量.vi" "版本号"() -> (w1158:string[])
    n728 = global read "从板全局变量.vi" "波特率"() -> (w1160:string[])
    n729 = global read "从板全局变量.vi" "满标志"() -> (w1166:dbl[])
    n730 = global read "从板全局变量.vi" "Life"() -> (w1163:dbl[])
    n731 = Index Array(array=w1163, index=w1101) -> (element=w1098:dbl)
    n732 = Index Array(array=w1160, index=w1101) -> (element=w1154:string)
    n733 = Index Array(array=w1161, index=w1101) -> (element=w1155:string)
    n734 = Index Array(array=w1164, index=w1101) -> (element=w1150:dbl)
    n735 = Index Array(array=w1166, index=w1101) -> (element=w1148:dbl)
    n736 = Index Array(array=w1157, index=w1101) -> (element=→"故障信息":string)
    n737 = Index Array(array=w1158, index=w1101) -> (element=w1152:string)
    n738 = Index Array(array=w1165, index=w1101) -> (element=w1149:dbl)
    n739 = Index Array(array=w1162, index=w1101) -> (element=w1156:string)
    n740 = Index Array(array=w1159, index=w1101) -> (element=w1153:string)
    n741 = local write "协议版本号"(w1152) -> ()
    n742 = local write "波特率"(w1154) -> ()
    n743 = local write "应用类型"(w1153) -> ()
    n744 = local write "协议是否公开"(w1155) -> ()
    n745 = local write "电池运行状态"(w1156) -> ()
    n746 = local write "Life:"(w1098) -> ()
    n747 = global read "中英文全局.vi" "中英文选择"() -> (w1095:enum32{"中文", "English"})
    n748 = case shown="\"中文\"" w1095 {
      tunnel: [w1220 w1225] -> w1196
      tunnel: w1148 -> [w1219 w1224]
      frame "English" {
        n749 = case shown="AA" w1219 {
          tunnel: [_ "Clean" "Charge,But not full" "Full"] -> w1220
          frame 0, Default {
          }
          frame 85 {
          }
          frame 90 {
          }
          frame 170 {
          }
        }
      }
      frame "中文" {
        n750 = case shown="5A" w1224 {
          tunnel: [_ "清除" "充电,但未充满" "充满"] -> w1225
          frame 0, Default {
          }
          frame 85 {
          }
          frame 90 {
          }
          frame 170 {
          }
        }
      }
    }
    n751 = call "各种状态子VI.vi"("颜色输入"=u32[] [16448250, 6618880, 16711680, 16860], "状态输入"=string[][] [["Close", "Open", "Fault", "Invalid"], ["Close", "Open", "Fault", "Invalid"], ["Close", "Open", "Fault", "Invalid"], ["Close", "Open", "Fault", "Invalid"]], "几种类型"=4, "数值"=w1150) -> ("状态"=w1193:string[])  [unwired: 1 out]
    n752 = call "各种状态子VI.vi"("颜色输入"=u32[] [16448250, 6618880, 16711680, 16860], "状态输入"=string[][] [["Close", "Open", "Fault", "Invalid"], ["Close", "Open", "Fault", "Invalid"], ["Close", "Open", "Fault", "Invalid"], ["Close", "Open", "Fault", "Invalid"]], "几种类型"=4, "数值"=w1149) -> ("状态"=w1194:string[])  [unwired: 1 out]
    n753 = local write "电池充满标志位"(w1196) -> ()
    n754 = Build Array(w1193, w1194) -> (w1195:string[][])
    n755 = Reshape Array(w1195, 8 ("维数大小")) -> (w1096:string[])
    n756 = local write "继电器状态"(w1096) -> ()
    n757 = global read "从板全局变量.vi" "F"() -> (w1103:dbl[][])
    n758 = global read "从板全局变量.vi" "故障信息"() -> (w1135:string[])
    n759 = Index Array(array=w1103, index (row)=w1101) -> (element=w1102:dbl[])  [unwired: 1 in]
    n760 = Index Array(array=w1135, index=w1101) -> (element=w1133:string)
    n761 = Index Array(array=w1102) -> (element #1=w1111:dbl, element #2=w1110:dbl, element #3=w1109:dbl, element #4=w1108:dbl, element #5=w1106:dbl, element #6=w1104:dbl)  [unwired: 6 in]
    n762 = for {
      N: 8 -> [_]
      tunnel: w1133 -> [w1274]
      tunnel: [w1269] -> w1132 mode=indexing
      i -> [w1273]
      w1271 = 2 ("x")
      n763 = Multiply(x=w1271, y=w1273) -> (x*y=w1272:i32)
      n764 = String Subset(string=w1274, offset (0)=w1272, length (rest)=w1271) -> (substring=w1270:string)
      n765 = Hexadecimal String To Number(string=w1270, default (0uL)=u8 0) -> (number=w1269:u8)  [unwired: 1 in, 1 out]
    }
    n766 = Format Into String(format string="%#f" ("格式字符串"), w1104) -> (resulting string=→"供电电源电压(V)":string)  [unwired: 2 in, 1 out]
    n767 = Format Into String(format string="%#f" ("格式字符串"), w1106) -> (resulting string=→"内网总线负载率":string)  [unwired: 2 in, 1 out]
    n768 = call "二进制解析-8.6.vi"("索引"=8, "数值"=w1110) -> ("低位子数组"=w1121:i32[])  [unwired: 3 out]
    n769 = call "二进制解析-8.6.vi"("索引"=8, "数值"=w1108) -> ("低位子数组"=w1114:i32[])  [unwired: 3 out]
    n770 = call "二进制解析-8.6.vi"("索引"=8, "数值"=w1111) -> ("低位子数组"=w1120:i32[])  [unwired: 3 out]
    n771 = call "二进制解析-8.6.vi"("索引"=8, "数值"=w1109) -> ("低位子数组"=w1115:i32[])  [unwired: 3 out]
    n772 = Index Array(array=w1132) -> (element #1=w1131:u8, element #2=w1130:u8, element #3=w1129:u8, element #4=w1128:u8, element #5=w1127:u8, element #6=w1126:u8, element #7=w1125:u8, element #8=w1124:u8)  [unwired: 8 in]
    n773 = for {
      N: 2 -> [_]
      tunnel: w1114 -> [w1234]
      i -> [w1232]
      w1236 = 2 ("y")
      n774 = Multiply(x=w1232, y=w1236) -> (x*y=w1235:i32)
      n775 = Array Subset(array=w1234, index=w1235, length=w1236) -> (w1233:i32[])
      n776 = call "数值二进制转十进制-8.6.vi"("子数组"=w1233) -> ("十进制数值"=w1231:i32)  [unwired: 4 out]
      n777 = case shown="1" w1232 {
        tunnel: w1231 -> [_ w1237 _ _]
        frame 0, Default {
        }
        frame 1 {
          "供电电源状态" <- w1237
        }
        frame 2 {
        }
        frame 3 {
        }
      }
    }
    n778 = for {
      N: 4 -> [_]
      tunnel: w1121 -> [w1251]
      i -> [w1249]
      w1253 = 2 ("y")
      n779 = Multiply(x=w1249, y=w1253) -> (x*y=w1252:i32)
      n780 = Array Subset(array=w1251, index=w1252, length=w1253) -> (w1250:i32[])
      n781 = call "数值二进制转十进制-8.6.vi"("子数组"=w1250) -> ("十进制数值"=w1248:i32)  [unwired: 4 out]
      n782 = case shown="3" w1249 {
        tunnel: w1248 -> [w1254 w1255 w1256 w1257]
        frame 0, Default {
          "绝缘检测模块状态" <- w1254
        }
        frame 1 {
          "电流模块模块状态" <- w1255
        }
        frame 2 {
          "电池充电均衡模块状态" <- w1256
        }
        frame 3 {
          "电池放电均衡模块状态" <- w1257
        }
      }
    }
    n783 = for {
      N: 4 -> [_]
      tunnel: w1120 -> [w1261]
      i -> [w1259]
      w1263 = 2 ("y")
      n784 = Multiply(x=w1259, y=w1263) -> (x*y=w1262:i32)
      n785 = Array Subset(array=w1261, index=w1262, length=w1263) -> (w1260:i32[])
      n786 = call "数值二进制转十进制-8.6.vi"("子数组"=w1260) -> ("十进制数值"=w1258:i32)  [unwired: 4 out]
      n787 = case shown="0, 默认" w1259 {
        tunnel: w1258 -> [w1264 w1265 w1266 w1267]
        frame 0, Default {
          "温度模块检测状态" <- w1264
        }
        frame 1 {
          "内部总电压检测模块状态" <- w1265
        }
        frame 2 {
          "外部总电压检测模块状态" <- w1266
        }
        frame 3 {
          "电压模块检测状态" <- w1267
        }
      }
    }
    n788 = for {
      N: 4 -> [_]
      tunnel: w1115 -> [w1241]
      i -> [w1239]
      w1243 = 2 ("y")
      n789 = Multiply(x=w1239, y=w1243) -> (x*y=w1242:i32)
      n790 = Array Subset(array=w1241, index=w1242, length=w1243) -> (w1240:i32[])
      n791 = call "数值二进制转十进制-8.6.vi"("子数组"=w1240) -> ("十进制数值"=w1238:i32)  [unwired: 4 out]
      n792 = case shown="2" w1239 {
        tunnel: w1238 -> [w1244 w1245 w1246 w1247]
        frame 0, Default {
          "系统时钟状态" <- w1244
        }
        frame 1 {
          "Flash存储器状态" <- w1245
        }
        frame 2 {
          "外部EE存储器状态" <- w1246
        }
        frame 3 {
          "内部EE存储器状态" <- w1247
        }
      }
    }
    n793 = call "故障数值解析.vi"("输入"=w1131) -> ("结果"=w1146:string[])  [unwired: 2 out]
    n794 = call "故障数值解析.vi"("输入"=w1130) -> ("结果"=w1145:string[])  [unwired: 2 out]
    n795 = call "故障数值解析.vi"("输入"=w1129) -> ("结果"=w1144:string[])  [unwired: 2 out]
    n796 = call "故障数值解析.vi"("输入"=w1128) -> ("结果"=w1140:string[])  [unwired: 2 out]
    n797 = call "故障数值解析.vi"("输入"=w1127) -> ("结果"=w1143:string[])  [unwired: 2 out]
    n798 = call "故障数值解析.vi"("输入"=w1126) -> ("结果"=w1142:string[])  [unwired: 2 out]
    n799 = call "故障数值解析.vi"("输入"=w1125) -> ("结果"=w1141:string[])  [unwired: 2 out]
    n800 = call "故障数值解析.vi"("输入"=w1124) -> ("结果"=w1139:string[])  [unwired: 2 out]
    n801 = Build Array(w1146, w1145, w1144, w1140, w1143, w1142, w1141, w1139) -> (w1137:string[][])
    n802 = Reshape Array(w1137, 32 ("维数大小")) -> (w1136:string[])
    n803 = case shown="\"English\"" w1095 {
      tunnel: [string[] ["电压检测模块故障", "温度检测模块故障", "电流检测模块故障", "绝缘检测模块故障", "内总电压检测模块故障", "外总电压检测模块故障", "系统外扩时钟模块故障", "CPU内部EE故障", "EE存储器故障", "45db041存储器故障", "CPU内部FLASH存储器故障", "CPU故障", "CAN4通信模块故障", "CAN0通信模块故障", "CAN1通信模块故障", "保留", "保留", "保留", "保留", "保留", "充电均衡模块故障", "放电均衡模块故障", "保留", "软件故障", "保留", "保留", "保留", "保留", "DI模块故障", "DO模块故障", "保留", "保留"] ("名称") string[] ["detection_cellv", "detection_temper", "detection_curr", "detection_iso", "detection_sumv_in", "detection_sumv_out", "detection_exterm_clock", "detection_ee_cpu", "detection_ee_ext", "detection_flash_ext", "detection_flash_cpu", "cpu_error", "detection_can4", "detection_can0", "detection_can1", "rsv", "rsv", "rsv", "rsv", "rsv", "detection_chg_bal", "detection_dch_bal", "rsv", "soft_error", "rsv", "rsv", "rsv", "rsv", "DI_error", "DO_error", "rsv", "rsv"] ("名称")] -> w1147
      frame "中文", Default {
      }
      frame "English" {
      }
    }
    n804 = call "故障分解.vi"("名称"=w1147, "故障输入口"=w1136) -> ("输出数组"=→"硬件故障":string[][])  [unwired: 1 in, 2 out]
  }
  n805 = local write "布尔 3"(TRUE ("布尔 3")) -> ()
  "单选选项2" <- FALSE ("单选选项2")
